vi "Grain Boundary Genie.vi"() -> ()   [LabVIEW 2010]
uses:
  <vilib>/Analysis/baseanly.llb/Real Dot Product.vi
  <vilib>/Analysis/baseanly.llb/Vector x A.vi
  <vilib>/Analysis/_algsub.llb/Real Vector Norm.vi
  <vilib>/Analysis/baseanly.llb/Real A x B.vi
  <vilib>/Utility/file.llb/Write To Spreadsheet File (string).vi
  <vilib>/Utility/file.llb/Read From Spreadsheet File (string).vi
  <vilib>/Analysis/NI_AALBase.lvlib
  <vilib>/Analysis/NI_AALPro.lvlib
  <vilib>/picture/3D Picture Control/NI_3D Picture Control.lvlib
  <vilib>/Analysis/baseanly.llb/A x Vector.vi
panel:
  in  "New Lattice Vector a 2":dbl[](array[numeric])=[6.0, 0.0, 0.0]
  in  "New Lattice Vector b 2":dbl[](array[numeric])=[0.0, 6.0, 0.0]
  in  "New Lattice Vector c 2":dbl[](array[numeric])=[0.0, 0.0, 6.0]
  out "Grain Boundary Definition":T1={"Grain 1 Orientation"=[1.0, 0.0, 0.0], "Grain 2 Orientation"=[1.0, 0.0, 0.0], "Twist Angle (Deg)"=0.0, "Translation Vector"=[0.0, 0.0, 0.0]}
  in  "Make GB":bool=TRUE
  out "STEM Viewing Angles Array":dbl[][](array[numeric])=[[0.0, 1.0, 0.0], [0.0, 0.0, 1.0], [0.0, 1.0, 1.0], [0.0, -1.0, 1.0], [0.0, 1.0, -1.0]]
  in  "Make Grain 2":bool=TRUE
  in  "Make Grain 1":bool=TRUE
  out "Grain 2 Primative":T2={"Structure Name"="CdTe", "Lattice vector a"=[0.0, 0.0, 6.615785553057252], "Lattice vector b"=[6.615785553057252, 0.0, 0.0], "Lattice vector c"=[0.0, -6.615785553057252, 0.0], "Atoms Array"=[{"Atom Name"="Cd", "Positions (Direct)"=[[0.0, 0.0, 0.0], [0.0, 0.5, 0.5], [0.5, 0.0, 0.5], [0.5, 0.5, 0.0]], "Positions (Cartesian)"=[[0.0, 0.0, 0.0], [3.307892776528626, -3.307892776528626, 0.0], [0.0, -3.307892776528626, 3.307892776528626], [3.307892776528626, 0.0, 3.307892776528626]]}, {"Atom Name"="Te", "Positions (Direct)"=[[0.25, 0.25, 0.25], [0.75, 0.75, 0.25], [0.75, 0.25, 0.75], [0.25, 0.75, 0.75]], "Positions (Cartesian)"=[[1.653946388264313, -1.653946388264313, 1.653946388264313], [4.96183916479294, -1.653946388264313, 4.96183916479294], [1.653946388264313, -4.96183916479294, 4.96183916479294], [4.96183916479294, -4.96183916479294, 1.653946388264313]]}], "# of atoms"=8} {"Atoms Array"."Positions (Cartesian)" format="%#_4f"; "Atoms Array"."Positions (Direct)" format="%#_4f"}
  in  "Load GB VESTA":bool
  in  "Load G2 VESTA":bool
  in  "Load G1 VESTA":bool
  in  "Conventional Unit Cell":T2={"Structure Name"="CdTe", "Lattice vector a"=[6.615785553057252, 0.0, 0.0], "Lattice vector b"=[0.0, 6.615785553057252, 0.0], "Lattice vector c"=[0.0, 0.0, 6.615785553057252], "Atoms Array"=[{"Atom Name"="Cd", "Positions (Direct)"=[[0.0, 0.0, 0.0], [0.0, 0.5, 0.5], [0.5, 0.0, 0.5], [0.5, 0.5, 0.0]], "Positions (Cartesian)"=[[0.0, 0.0, 0.0], [0.0, 3.307892776528626, 3.307892776528626], [3.307892776528626, 0.0, 3.307892776528626], [3.307892776528626, 3.307892776528626, 0.0]]}, {"Atom Name"="Te", "Positions (Direct)"=[[0.25, 0.25, 0.25], [0.75, 0.75, 0.25], [0.75, 0.25, 0.75], [0.25, 0.75, 0.75]], "Positions (Cartesian)"=[[1.653946388264313, 1.653946388264313, 1.653946388264313], [4.96183916479294, 4.96183916479294, 1.653946388264313], [4.96183916479294, 1.653946388264313, 4.96183916479294], [1.653946388264313, 4.96183916479294, 4.96183916479294]]}], "# of atoms"=8}
  in  "Overlap Region":dbl(slide) scale=-2.0..2.0
  in  "Tab Control":T3(tab)
  in  "GB Slider":u16(ring) items=["G1 Height", "G1 Width", "G1 Length", "G1 Start"]
  in  "GB Size Slider":dbl(slide) scale=0.0..1.0
  in  "Suggest Sizes":bool
  in  "Integer Tolerance":dbl=0.01
  in  "GB Geometric Type":T4(tab)
  in  "Use same H and W":bool=TRUE
  in  "Grain 2 Size":T5={"Height"=1.0, "Width"=1.0, "Length"=1.0, "Start"=0.0}
  in  "Grain 1 Size":T5={"Height"=1.0, "Width"=1.0, "Length"=1.0, "Start"=0.0}
  in  "Grain 2 Monoclinic size":T6={"Height"=1.0, "Width"=1.0, "Angle (deg)"=1.0, "Length"=1.0, "Start"=0.0}
  in  "Grain 1 Monoclinic size":T6={"Height"=1.0, "Width"=1.0, "Angle (deg)"=1.0, "Length"=1.0, "Start"=0.0}
  in  "Use same H, W and angle":bool=TRUE
  in  "New Lattice Vector a":dbl[](array[numeric])=[6.0, 0.0, 0.0]
  in  "New Lattice Vector c":dbl[](array[numeric])=[0.0, 0.0, 6.0]
  in  "New Lattice Vector b":dbl[](array[numeric])=[0.0, 6.0, 0.0]
  in  "Options":cluster{"Border?":bool, "Bonds?":bool}={"Border?"=TRUE, "Bonds?"=FALSE}
  in  "Zoom Scale":dbl(slide)=0.06161137440758294 scale=0.0..0.2
  in  "Mutual Viewing Angle":dbl[](array[numeric])=[0.0, 1.0, 0.0]
  in  "STEM Viewing Angles":u16(ring) items=["[0,0,1]", "[-0,-0,-1]", "[-0,0,1]", "[0,-0,1]", "[0,0,-1]", "[-0,-0,1]", "[0,-0,-1]", "[-0,0,-1]", "[-1,1,0]", "[1,-1,0]", "[1,-1,-0]", "[-1,1,-0]"]
  in  "Setup Camera":bool
  out "STEM Viewable?":bool=TRUE
  in  "Force Orthorhombic?":bool
  in  "Remove Close Atoms":bool
  in  "Crop to Smallest Repeating":bool
  in  "Slab Y":dbl=6.0
  in  "Slab X":dbl=6.0
  in  "Tolerance (A)":dbl=1.0
  in  "Minimally Allowable Distance (A)":dbl=1.5
  out "# of Atoms Removed":i32
  out "Repeating X Length Scale":dbl=99.01964045547014
  out "Subset for X?":bool
  out "Repeating Y Length Scale":dbl=99.01964045547014
  out "Subset for Y?":bool
  out "% of normal atomic density":dbl=225.0005167366452
  out "Grain 2 Integers":dbl[](array[numeric])=[1.0, 1.0, 1.0]
  out "Grain 1 Integers":dbl[](array[numeric])=[1.0, 1.0, 1.0]
  out "Misorientation Angle":dbl=60.00000000000001
  out "Suggested Viewing Angle":dbl[](array[numeric])=[-1.0, 1.0, 0.0]
  out "# of Atoms":i32=36
  out "# of Cd Atoms":i32=28
  out "# of Te Atoms":i32=8
  in  "Load GB Config":bool
  in  "Save to GB config file":bool
  in  "Structure Name":string="(60.00) twist [1.000,1.000,1.000] [1.000,1.000,1.000] (0.00,0.00,0.00)T GB"
  in  "Save to POSCAR":bool
  in  "Relaxation Type":string(combo)="conv opti"
  in  "Save into GULP":bool
  in  "Vesta .exe Location":path=path "C:/Program Files (x86)/VESTA/VESTA.exe"
  out "Lattice Parameter":dbl=6.615785553057252
  in  "Timeout Activity":string(combo)="Analyze GB"
  out "Grain Boundary Object":refnum<vi>
  out "Grain 2 Object":refnum<vi>
  out "Grain 1 Object":refnum<vi>
  in  "Add Tilt Angle":dbl(slide) scale=-5.0..15.0
  out "Grain Boundary":T2={"Structure Name"="Grain Boundary", "Lattice vector a"=[6.615785553057252, 0.0, 0.0], "Lattice vector b"=[0.0, 6.615785553057252, 0.0], "Lattice vector c"=[0.0, 0.0, 13.231571106114504], "Atoms Array"=[{"Atom Name"="Cd", "Positions (Direct)"=[[0.0, 0.0, 0.0], [0.0, 0.0, 0.5], [0.0, 0.5, 0.25], [0.0, 1.0, 0.0], [0.0, 1.0, 0.5], [0.5, 0.0, 0.25], [0.5, 0.5, 0.0], [0.5, 0.5, 0.5], [0.5, 1.0, 0.25], [1.0, 0.0, 0.0], [1.0, 0.0, 0.5], [1.0, 0.5, 0.25], [1.0, 1.0, 0.0], [1.0, 1.0, 0.5], [0.0, 0.0, 0.5], [0.0, 0.0, 1.0], [0.0, 0.5, 0.75], [0.0, 1.0, 0.5], [0.0, 1.0, 1.0], [0.5, 0.0, 0.75], [0.5, 0.5, 0.5], [0.5, 0.5, 1.0], [0.5, 1.0, 0.75], [1.0, 0.0, 0.5], [1.0, 0.0, 1.0], [1.0, 0.5, 0.75], [1.0, 1.0, 0.5], [1.0, 1.0, 1.0]], "Positions (Cartesian)"=[[0.0, 0.0, 0.0], [0.0, 0.0, 6.615785553057252], [0.0, 3.307892776528626, 3.307892776528626], [0.0, 6.615785553057252, 0.0], [0.0, 6.615785553057252, 6.615785553057252], [3.307892776528626, 0.0, 3.307892776528626], [3.307892776528626, 3.307892776528626, 0.0], [3.307892776528626, 3.307892776528626, 6.615785553057252], [3.307892776528626, 6.615785553057252, 3.307892776528626], [6.615785553057252, 0.0, 0.0], [6.615785553057252, 0.0, 6.615785553057252], [6.615785553057252, 3.307892776528626, 3.307892776528626], [6.615785553057252, 6.615785553057252, 0.0], [6.615785553057252, 6.615785553057252, 6.615785553057252], [0.0, 0.0, 6.615785553057252], [0.0, 0.0, 13.231571106114504], [0.0, 3.307892776528626, 9.92367832958588], [0.0, 6.615785553057252, 6.615785553057252], [0.0, 6.615785553057252, 13.231571106114504], [3.307892776528626, 0.0, 9.92367832958588], [3.307892776528626, 3.307892776528626, 6.615785553057252], [3.307892776528626, 3.307892776528626, 13.231571106114504], [3.307892776528626, 6.615785553057252, 9.92367832958588], [6.615785553057252, 0.0, 6.615785553057252], [6.615785553057252, 0.0, 13.231571106114504], [6.615785553057252, 3.307892776528626, 9.92367832958588], [6.615785553057252, 6.615785553057252, 6.615785553057252], [6.615785553057252, 6.615785553057252, 13.231571106114504]]}, {"Atom Name"="Te", "Positions (Direct)"=[[0.25, 0.24999999999999992, 0.375], [0.25, 0.75, 0.125], [0.75, 0.24999999999999992, 0.125], [0.75, 0.75, 0.375], [0.25, 0.24999999999999992, 0.875], [0.25, 0.75, 0.625], [0.75, 0.24999999999999992, 0.625], [0.75, 0.75, 0.875]], "Positions (Cartesian)"=[[1.653946388264313, 1.6539463882643126, 4.96183916479294], [1.653946388264313, 4.96183916479294, 1.653946388264313], [4.96183916479294, 1.6539463882643126, 1.653946388264313], [4.96183916479294, 4.96183916479294, 4.96183916479294], [1.653946388264313, 1.6539463882643126, 11.577624717850192], [1.653946388264313, 4.96183916479294, 8.269731941321565], [4.96183916479294, 1.6539463882643126, 8.269731941321565], [4.96183916479294, 4.96183916479294, 11.577624717850192]]}], "# of atoms"=36} {"Atoms Array"."Positions (Cartesian)" format="%#_4f"; "Atoms Array"."Positions (Direct)" format="%#_4f"}
  out "Grain 2":T2={"Structure Name"="CdTe Expanded to Box", "Lattice vector a"=[6.615785553057252, 0.0, 0.0], "Lattice vector b"=[0.0, 6.615785553057252, 0.0], "Lattice vector c"=[0.0, 0.0, 6.615785553057252], "Atoms Array"=[{"Atom Name"="Cd", "Positions (Direct)"=[[0.0, 0.0, 0.0], [0.0, 0.0, 1.0], [0.0, 0.5, 0.5], [0.0, 1.0, 0.0], [0.0, 1.0, 1.0], [0.5, 0.0, 0.5], [0.5, 0.5, 0.0], [0.5, 0.5, 1.0], [0.5, 1.0, 0.5], [1.0, 0.0, 0.0], [1.0, 0.0, 1.0], [1.0, 0.5, 0.5], [1.0, 1.0, 0.0], [1.0, 1.0, 1.0]], "Positions (Cartesian)"=[[0.0, 0.0, 0.0], [0.0, 0.0, 6.615785553057252], [0.0, 3.307892776528626, 3.307892776528626], [0.0, 6.615785553057252, 0.0], [0.0, 6.615785553057252, 6.615785553057252], [3.307892776528626, 0.0, 3.307892776528626], [3.307892776528626, 3.307892776528626, 0.0], [3.307892776528626, 3.307892776528626, 6.615785553057252], [3.307892776528626, 6.615785553057252, 3.307892776528626], [6.615785553057252, 0.0, 0.0], [6.615785553057252, 0.0, 6.615785553057252], [6.615785553057252, 3.307892776528626, 3.307892776528626], [6.615785553057252, 6.615785553057252, 0.0], [6.615785553057252, 6.615785553057252, 6.615785553057252]]}, {"Atom Name"="Te", "Positions (Direct)"=[[0.25, 0.24999999999999992, 0.75], [0.25, 0.75, 0.25], [0.75, 0.24999999999999992, 0.25], [0.75, 0.75, 0.75]], "Positions (Cartesian)"=[[1.653946388264313, 1.6539463882643126, 4.96183916479294], [1.653946388264313, 4.96183916479294, 1.653946388264313], [4.96183916479294, 1.6539463882643126, 1.653946388264313], [4.96183916479294, 4.96183916479294, 4.96183916479294]]}], "# of atoms"=18} {"Atoms Array"."Positions (Cartesian)" format="%#_4f"; "Atoms Array"."Positions (Direct)" format="%#_4f"}
  out "Grain 1":T2={"Structure Name"="CdTe Expanded to Box", "Lattice vector a"=[6.615785553057252, 0.0, 0.0], "Lattice vector b"=[0.0, 6.615785553057252, 0.0], "Lattice vector c"=[0.0, 0.0, 6.615785553057252], "Atoms Array"=[{"Atom Name"="Cd", "Positions (Direct)"=[[0.0, 0.0, 0.0], [0.0, 0.0, 1.0], [0.0, 0.5, 0.5], [0.0, 1.0, 0.0], [0.0, 1.0, 1.0], [0.5, 0.0, 0.5], [0.5, 0.5, 0.0], [0.5, 0.5, 1.0], [0.5, 1.0, 0.5], [1.0, 0.0, 0.0], [1.0, 0.0, 1.0], [1.0, 0.5, 0.5], [1.0, 1.0, 0.0], [1.0, 1.0, 1.0]], "Positions (Cartesian)"=[[0.0, 0.0, 0.0], [0.0, 0.0, 6.615785553057252], [0.0, 3.307892776528626, 3.307892776528626], [0.0, 6.615785553057252, 0.0], [0.0, 6.615785553057252, 6.615785553057252], [3.307892776528626, 0.0, 3.307892776528626], [3.307892776528626, 3.307892776528626, 0.0], [3.307892776528626, 3.307892776528626, 6.615785553057252], [3.307892776528626, 6.615785553057252, 3.307892776528626], [6.615785553057252, 0.0, 0.0], [6.615785553057252, 0.0, 6.615785553057252], [6.615785553057252, 3.307892776528626, 3.307892776528626], [6.615785553057252, 6.615785553057252, 0.0], [6.615785553057252, 6.615785553057252, 6.615785553057252]]}, {"Atom Name"="Te", "Positions (Direct)"=[[0.25, 0.24999999999999992, 0.75], [0.25, 0.75, 0.25], [0.75, 0.24999999999999992, 0.25], [0.75, 0.75, 0.75]], "Positions (Cartesian)"=[[1.653946388264313, 1.6539463882643126, 4.96183916479294], [1.653946388264313, 4.96183916479294, 1.653946388264313], [4.96183916479294, 1.6539463882643126, 1.653946388264313], [4.96183916479294, 4.96183916479294, 4.96183916479294]]}], "# of atoms"=18} {"Atoms Array"."Positions (Cartesian)" format="%#_4f"; "Atoms Array"."Positions (Direct)" format="%#_4f"}
  in  "Primitive Lattice Vectors":T2={"Structure Name"="Relax2 Subcrystal", "Lattice vector a"=[0.0, 3.3046962263585, 3.3046962263585], "Lattice vector b"=[3.3046962263585, 0.0, 3.3046962263585], "Lattice vector c"=[3.3046962263585, 3.3046962263585, 0.0], "Atoms Array"=[{"Atom Name"="Cd", "Positions (Direct)"=[[0.0, 0.0, 0.0]], "Positions (Cartesian)"=[[0.0, 0.0, 0.0]]}, {"Atom Name"="Te", "Positions (Direct)"=[[0.25, 0.25, 0.25]], "Positions (Cartesian)"=[[1.65234811317925, 1.65234811317925, 1.65234811317925]]}], "# of atoms"=2} {"Atoms Array"."Positions (Cartesian)" format="%#_4f"; "Atoms Array"."Positions (Direct)" format="%#_4f"}
  out "Grain Boundary Render":refnum<vi>(3d-picture)
  in  "Translation Vector":dbl[](array[slide])=[0.0, 0.0, 0.0] scale=0.0..4.0
  in  "Twist Angle":dbl(slide) scale=0.0..38.0
  in  "Grain 2 Orientation":dbl[](array[numeric])=[1.0, 0.0, 0.0]
  in  "Grain 1 Orientation":dbl[](array[numeric])=[1.0, 0.0, 0.0]
  out "Grain 2 Render":refnum<vi>(3d-picture)
  out "Grain 1 Render":refnum<vi>(3d-picture)
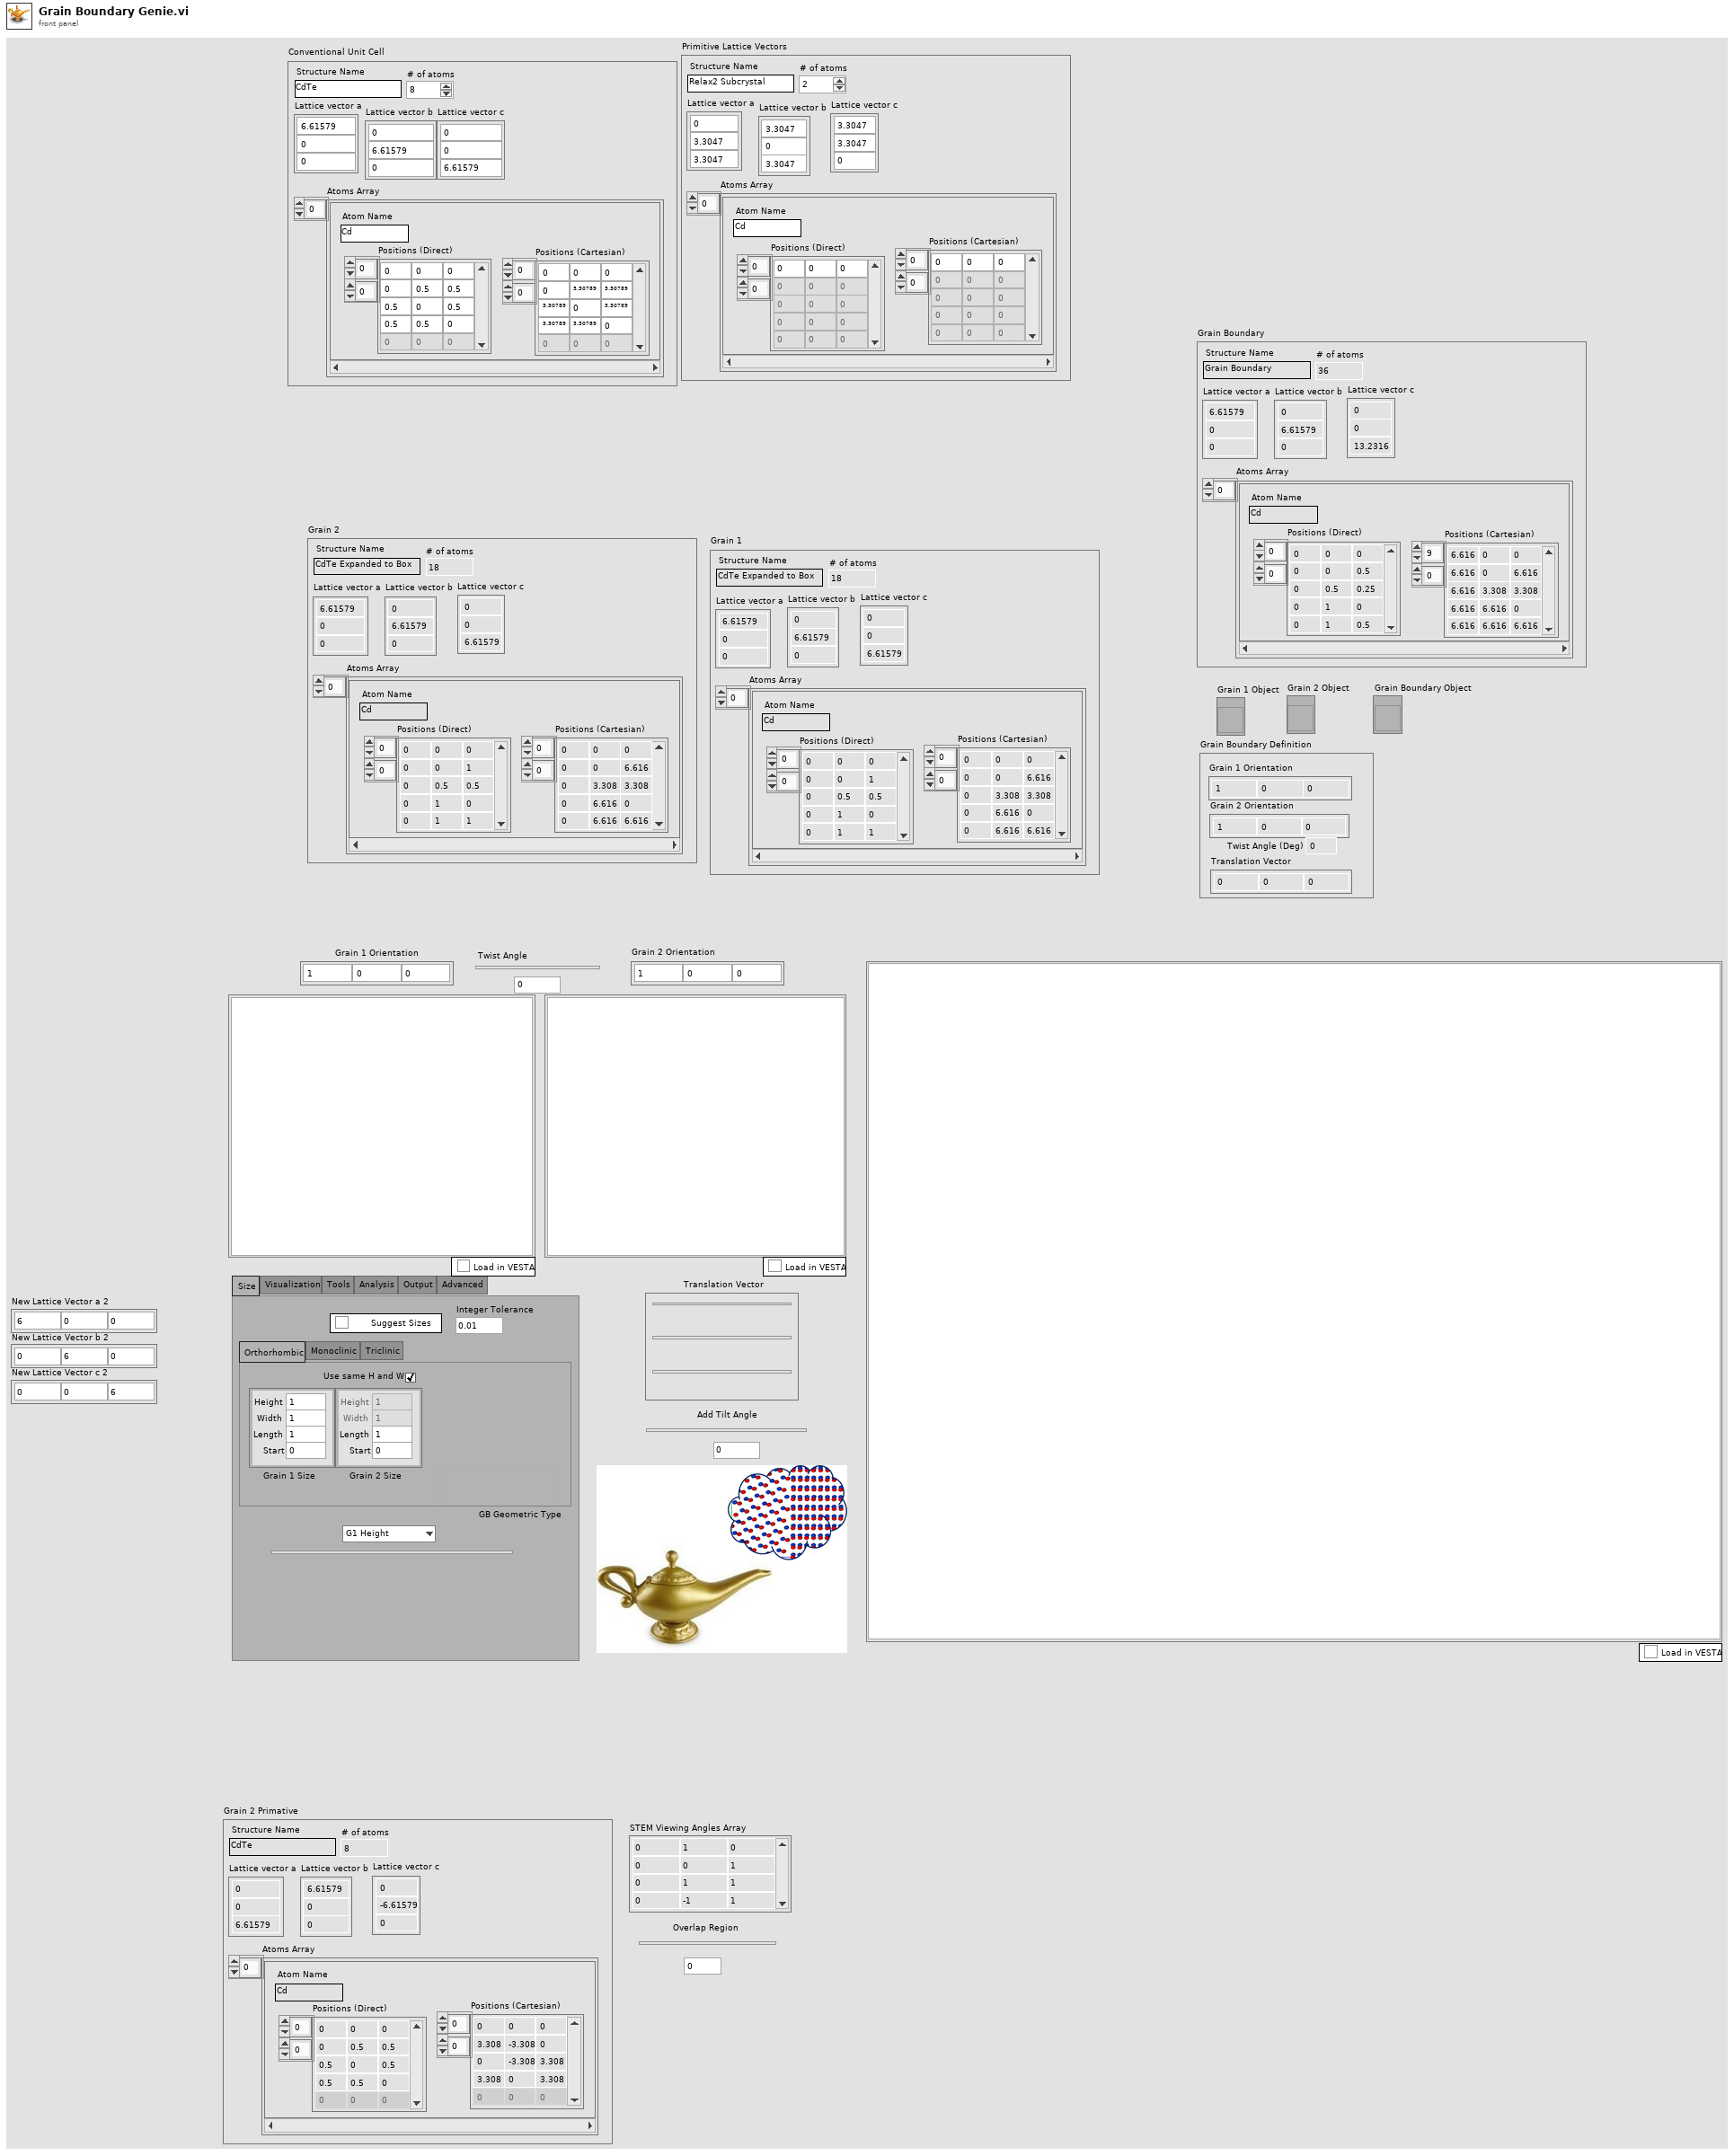
[diagram p1: front panel]
types:
  T1 = cluster{"Grain 1 Orientation":dbl[], "Grain 2 Orientation":dbl[], "Twist Angle (Deg)":dbl, "Translation Vector":dbl[]}
  T2 = cluster{"Structure Name":string, "Lattice vector a":dbl[], "Lattice vector b":dbl[], "Lattice vector c":dbl[], "Atoms Array":cluster{"Atom Name":string, "Positions (Direct)":dbl[][], "Positions (Cartesian)":dbl[][]}[], "# of atoms":i32}
  T3 = enum32{"Size", "Visualization", "Tools", "Analysis", "Output", "Advanced"}
  T4 = enum32{"Orthorhombic", "Monoclinic", "Triclinic"}
  T5 = cluster{"Height":dbl, "Width":dbl, "Length":dbl, "Start":dbl}
  T6 = cluster{"Height":dbl, "Width":dbl, "Angle (deg)":dbl, "Length":dbl, "Start":dbl}
  T7 = enum8{"Enabled", "Disabled", "Disabled and Grayed Out"}
  T8 = cluster{"Atom Name":string, "Positions (Direct)":dbl[][], "Positions (Cartesian)":dbl[][]}[]
  T9 = typedef "NI_Matrix.lvlib/RealMatrix.ctl" = dbl[][]
  T10 = cluster{"Misorientation Angle":dbl, "Misorientation Axis, o":dbl[], "Misorientation Matrix":T9}
  T11 = cluster{"Atom Name":string, "Positions (Direct)":dbl[][], "Positions (Cartesian)":dbl[][]}
  T12 = cluster{"Grain 1 Orientation":dbl[], "Grain 2 Orientation":dbl[], "Twist Angle":dbl, "Translation Vector":dbl[]}
  T13 = cluster{"Z Min":dbl, "Width":dbl, "Z Min":dbl, "Height":dbl, "Start":dbl, "Length":dbl}
  T14 = cluster{"Z Min":dbl, dbl, "Z Min":dbl, dbl, "Start":dbl, "Length":dbl}
  T15 = cluster{"Z Min":dbl, dbl, "Z Min":dbl, dbl, "Z Min":dbl, dbl}
  T16 = cluster{"Z Min":dbl, "Width":dbl, "Z Min":dbl, dbl, "Start":dbl, "Length":dbl}
  T17 = cluster{"String":dbl, "String":dbl, "String":dbl, "String":dbl}
  T18 = cluster{"Grain 1 Orientation":dbl[], "Grain 2 Orientation":dbl[], "Twist Angle":dbl}
  T19 = cluster{"Grain 1 Length (prop)":dbl, "Grain 2 Length (prop)":dbl, "Grain 1 Height (prop)":dbl, "Grain 2 Height (prop)":dbl, "Grain 1 Width (prop)":dbl, "Grain 2 Width (prop)":dbl}
  T20 = cluster{"Grain 1 Height (prop)":dbl, "Grain 1 Width (prop)":dbl, "Grain 1 Length (prop)":dbl, "y":dbl}
  T21 = cluster{"Grain 2 Height (prop)":dbl, "Grain 2 Width (prop)":dbl, "Grain 2 Length (prop)":dbl, "y":dbl}
  T22 = cluster{"[0]":dbl, "[1]":dbl, "[2]":dbl, "[3]":dbl}
  T23 = cluster{"[0]":dbl, "[1]":dbl, "[2]":dbl, "[3]":dbl, "[4]":dbl}
  T24 = cluster{"Lattice vector b[0]":dbl, "Lattice vector b[1]":dbl, "Lattice vector b[2]":dbl}
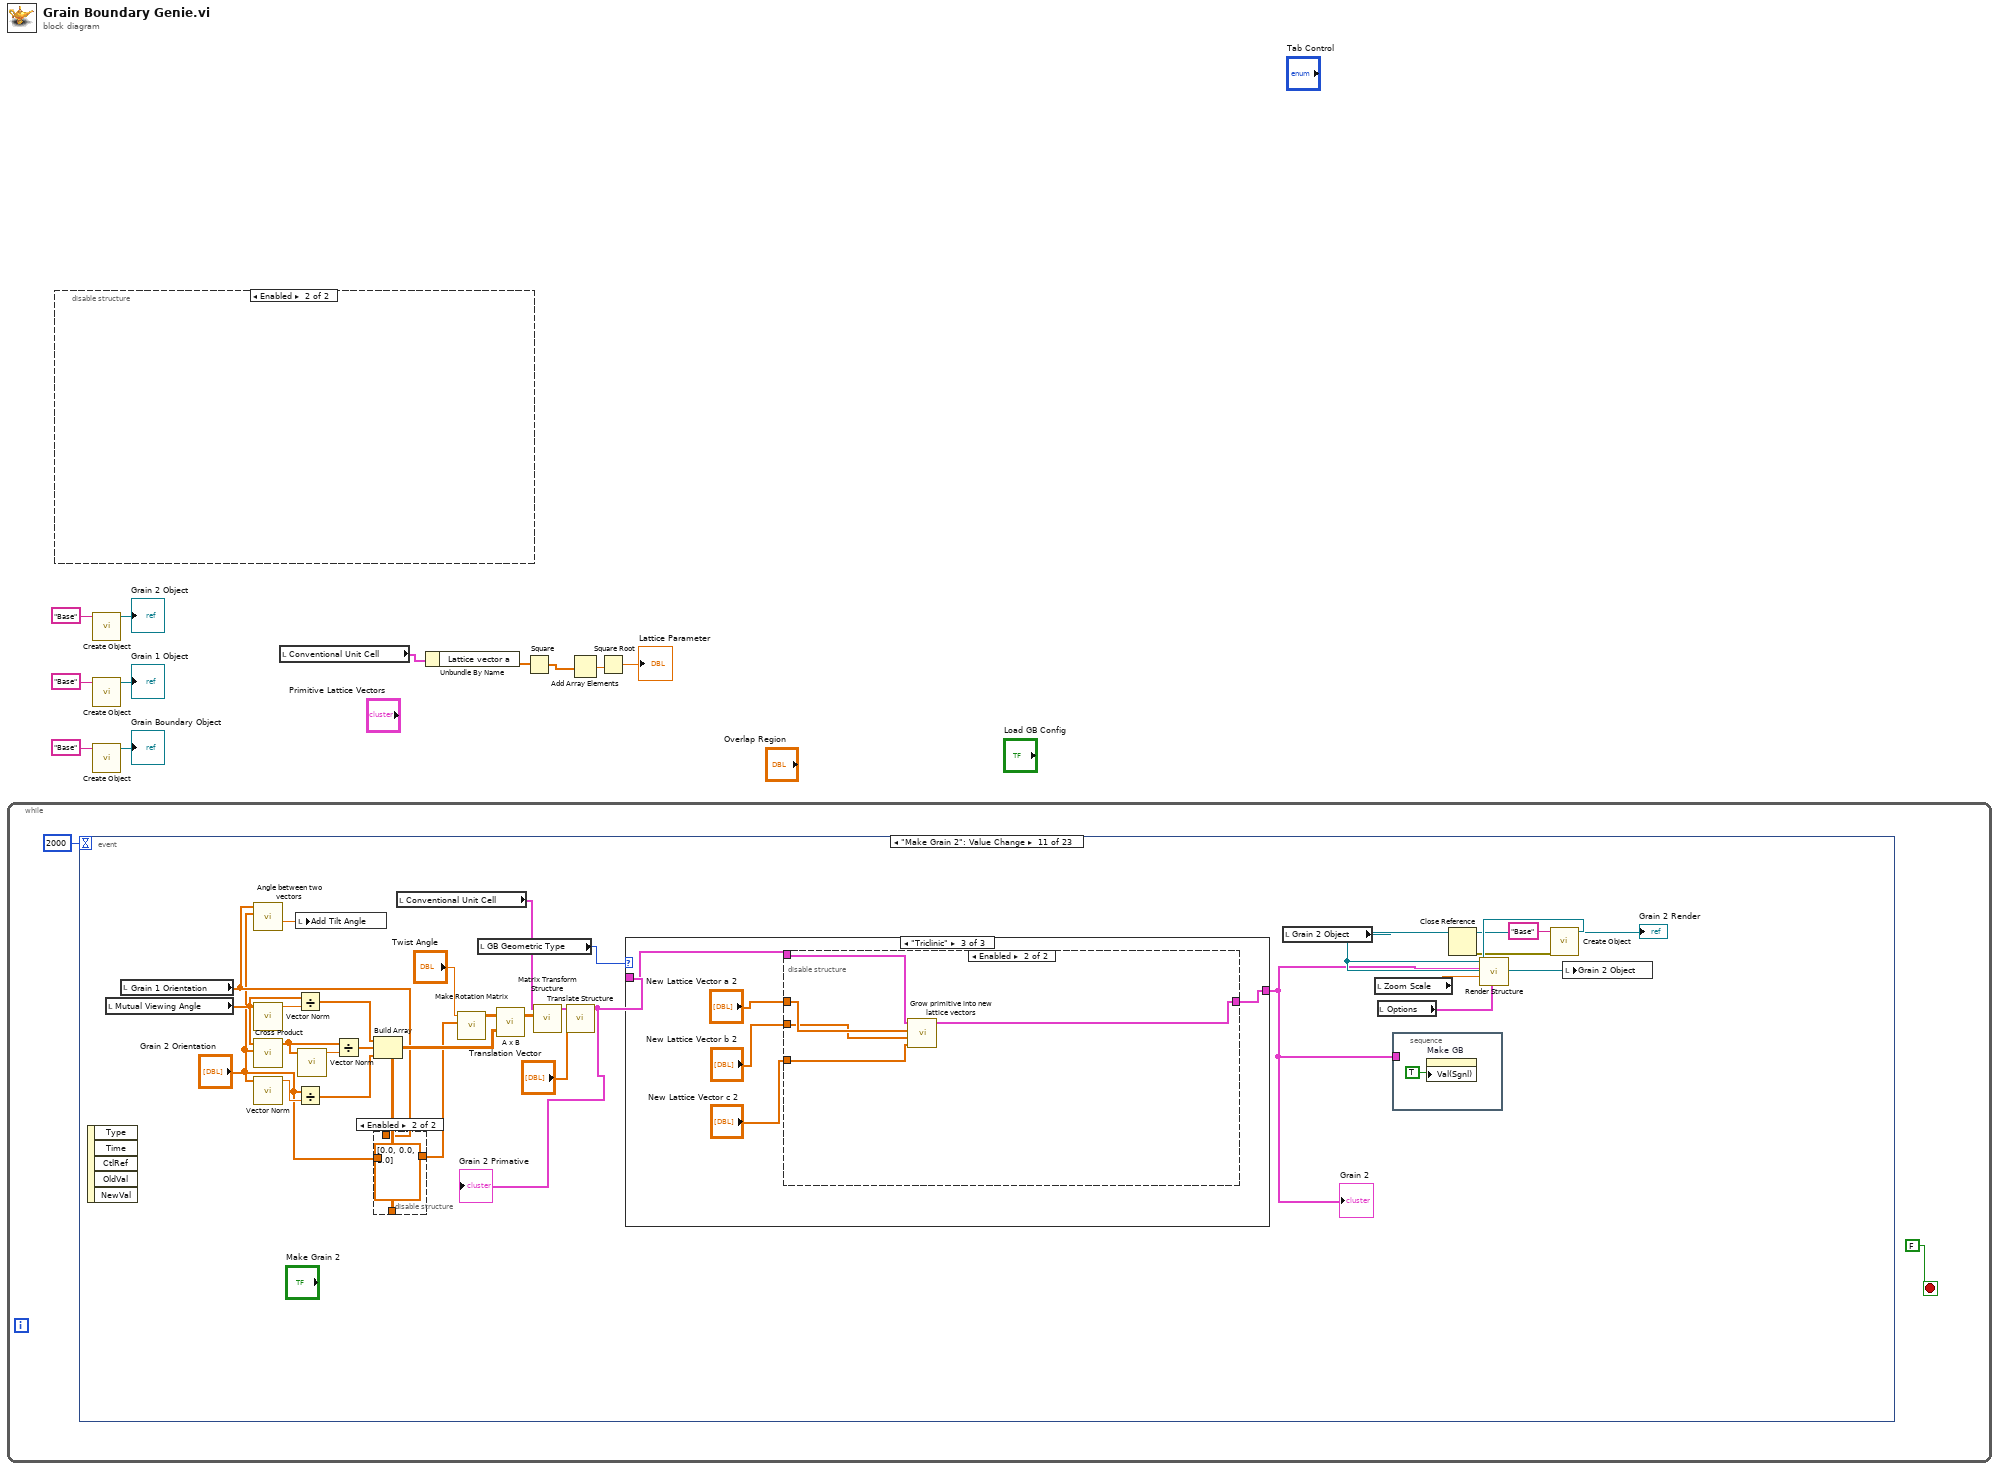
[diagram p0: block diagram]
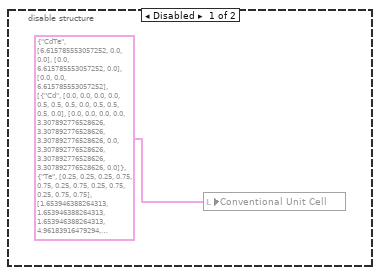
[diagram p2: hidden frame]
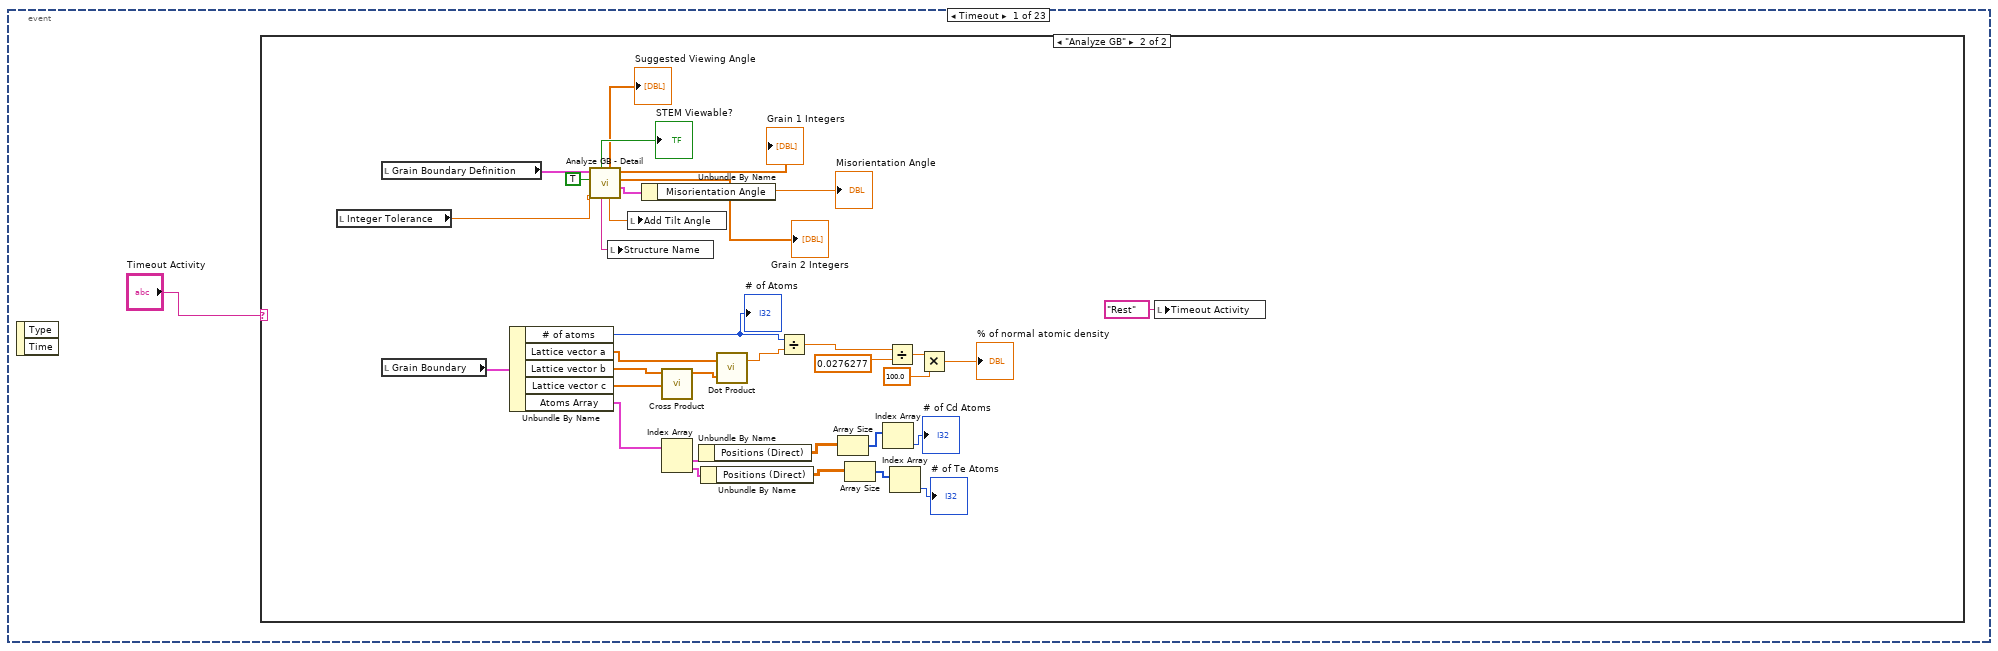
[diagram p3: hidden frame]
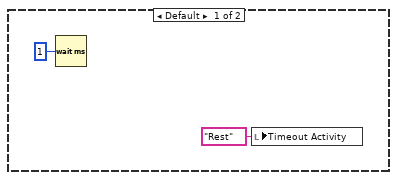
[diagram p4: hidden frame]
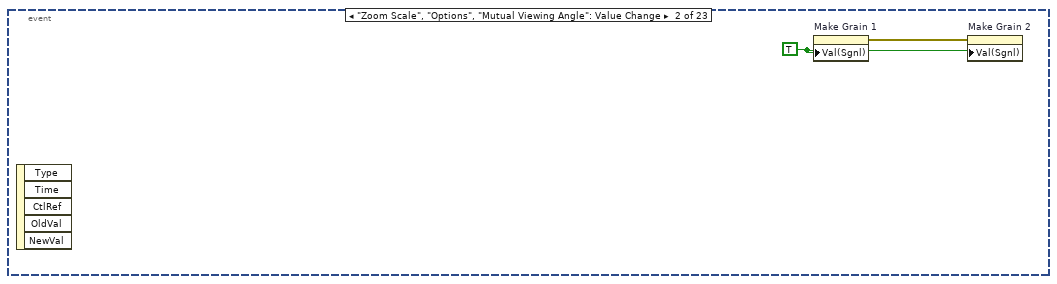
[diagram p5: hidden frame]
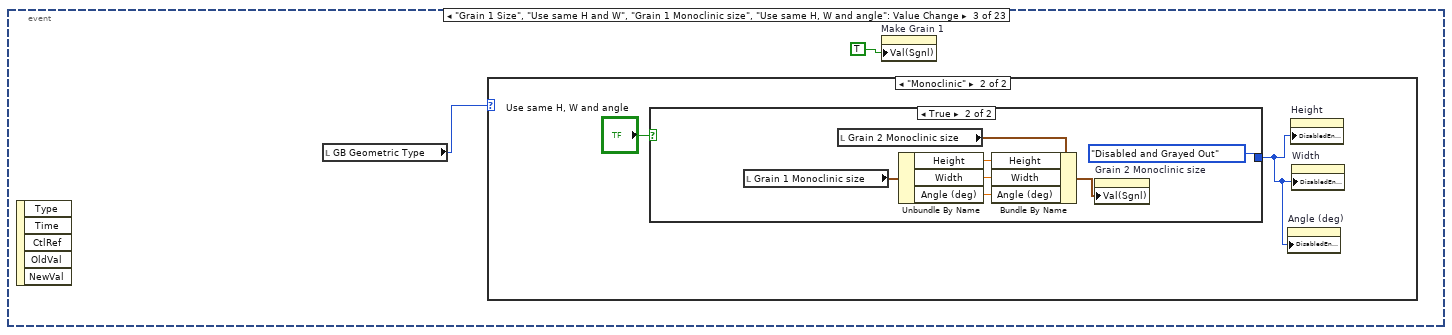
[diagram p6: hidden frame]
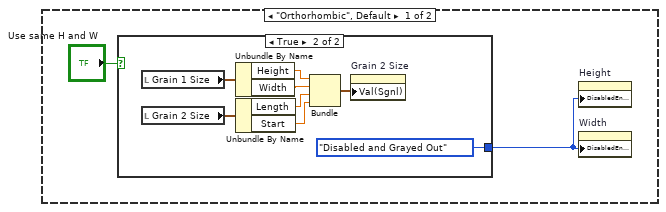
[diagram p7: hidden frame]
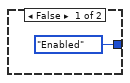
[diagram p8: hidden frame]
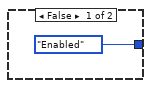
[diagram p9: hidden frame]
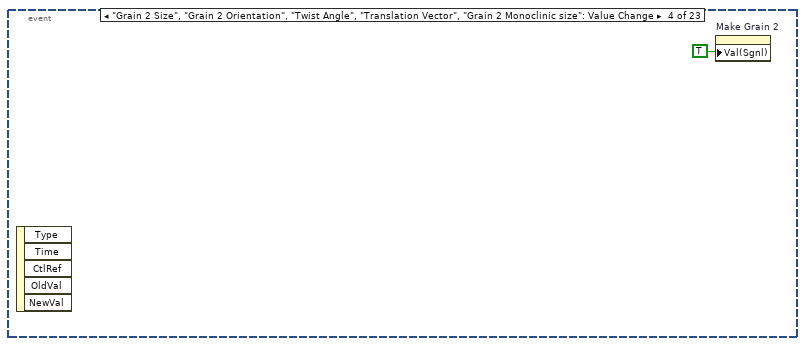
[diagram p10: hidden frame]
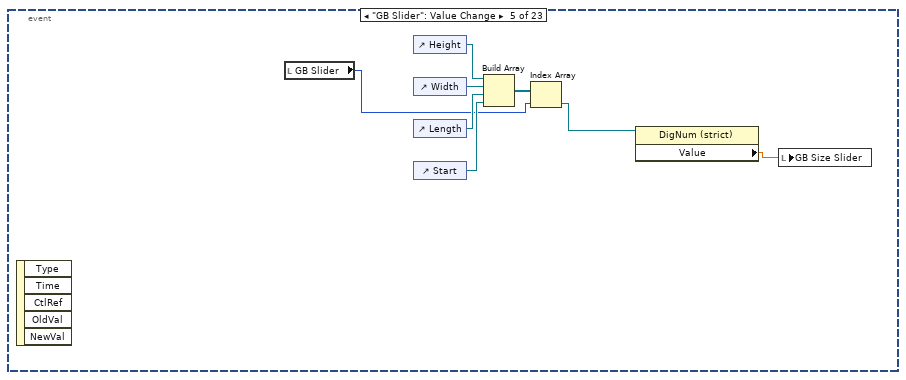
[diagram p11: hidden frame]
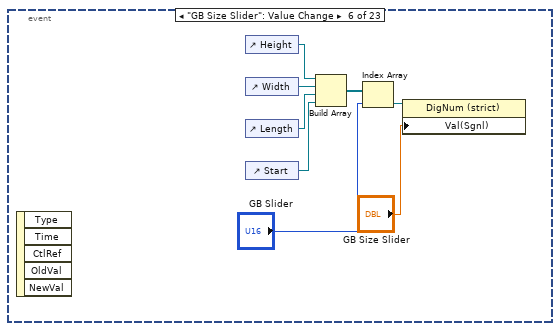
[diagram p12: hidden frame]
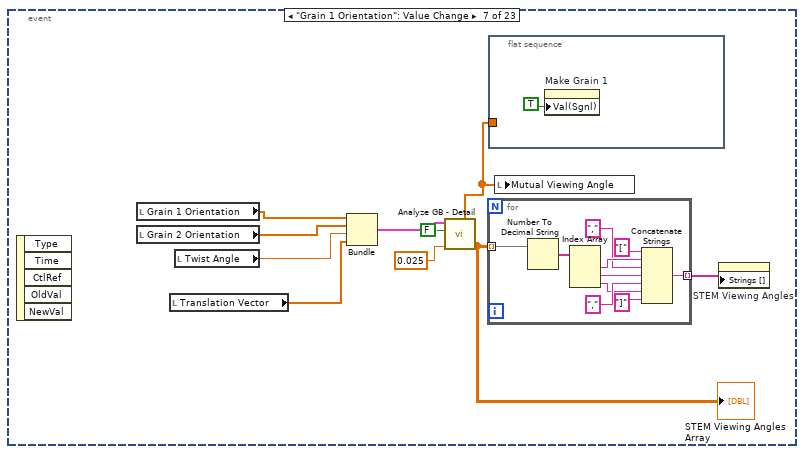
[diagram p13: hidden frame]
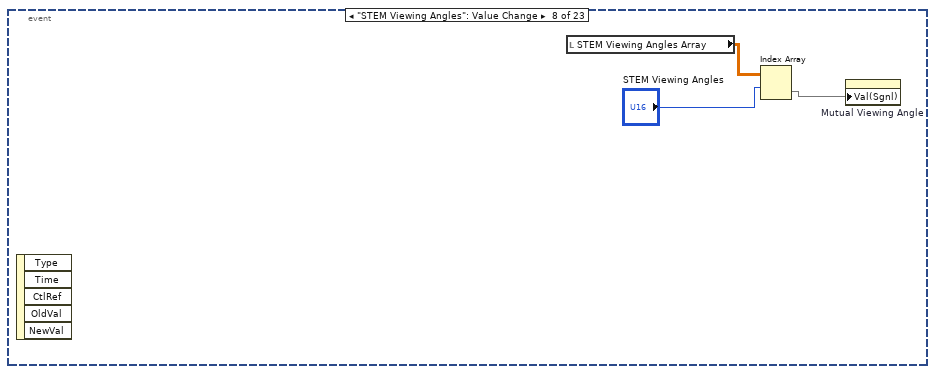
[diagram p14: hidden frame]
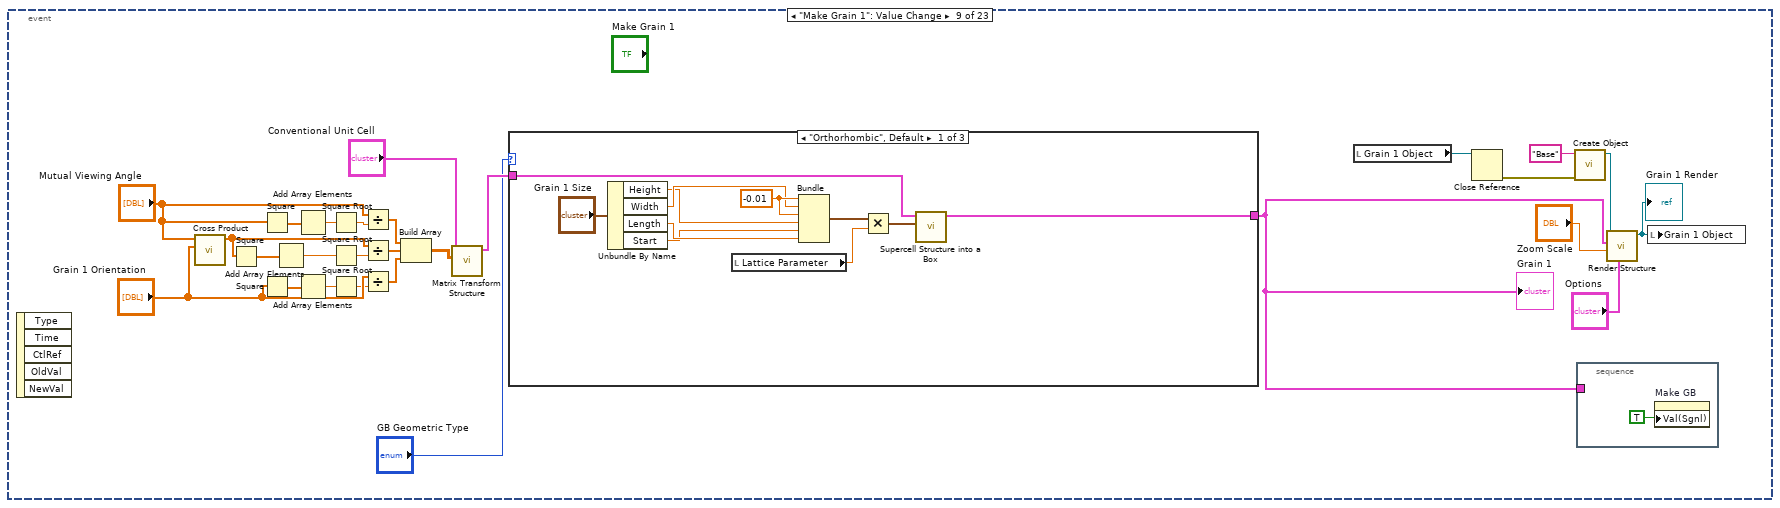
[diagram p15: hidden frame]
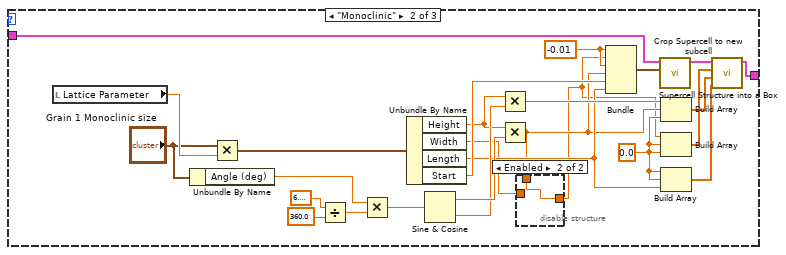
[diagram p16: hidden frame]
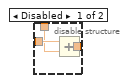
[diagram p17: hidden frame]
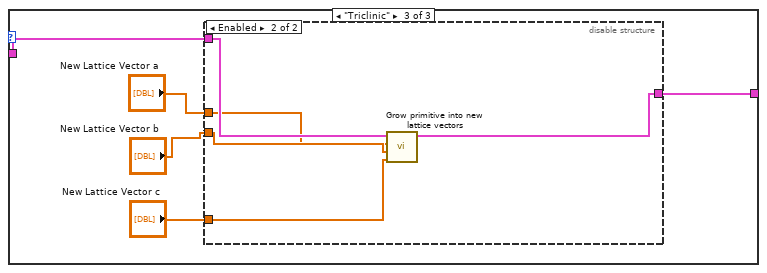
[diagram p18: hidden frame]
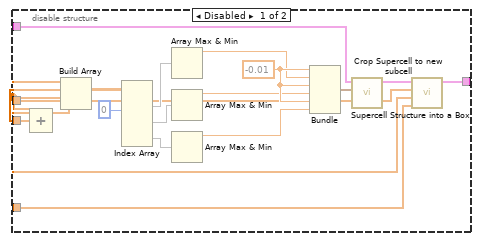
[diagram p19: hidden frame]
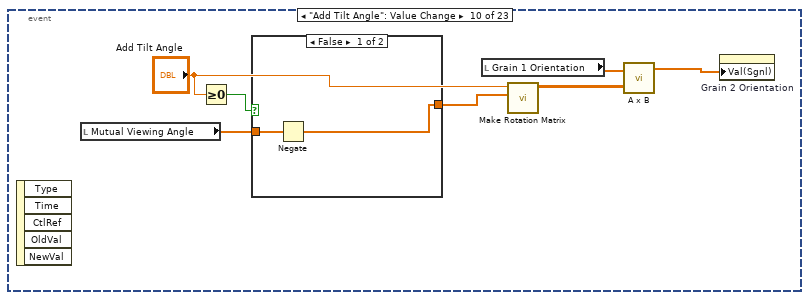
[diagram p20: hidden frame]
diagram:
  n1 = while {
    stop <- FALSE stop-if-true
    n2 = event shown="[10] \"Make Grain 2\": Value Change" {
      selector: _ -> [_ _ _ _ _ _ _ _ _ _ _ _ _ _ _ _ _ _ _ _ _ _ _]
      dyn-events: _ -> [_ _ _ _ _ _ _ _ _ _ _ _ _ _ _ _ _ _ _ _ _ _ _]
      timeout: 2000 -> [_ _ _ _ _ _ _ _ _ _ _ _ _ _ _ _ _ _ _ _ _ _ _]
      event Timeout {
        n3 = event-data() -> ()  [unwired: 1 in, 2 out]
        n4 = case shown="\"Analyze GB\"" "Timeout Activity" {
          frame Default {
            n5 = Wait (ms)(milliseconds to wait=u32 1) -> ()  [unwired: 1 out]
            n6 = local write "Timeout Activity"("Rest" ("Timeout Activity")) -> ()
          }
          frame "Analyze GB" {
            n7 = local read "Integer Tolerance"() -> (w21:dbl)
            n8 = local read "Grain Boundary Definition"() -> (w49:T1)
            n9 = local read "Grain Boundary"() -> (w23:T2)
            n10 = Unbundle By Name(w23) -> ("# of atoms"=w24:i32, "Lattice vector a"=w31:dbl[], "Lattice vector b"=w30:dbl[], "Lattice vector c"=w29:dbl[], "Atoms Array"=w22:T8)
            "# of Atoms" <- w24
            n11 = call "Analyze GB - Detail.vi"("Integer Tolerance"=w21, "Find Integer Rep?"=TRUE, "Grain Boundary Definition"=w49) -> ("Misorientation"=w35:T10, "Grain 2 Integers"=→"Grain 2 Integers":dbl[], "Grain 1 Integers"=→"Grain 1 Integers":dbl[], "Tilt Angle (Deg)"=w38:dbl, "Suggested view direction"=→"Suggested Viewing Angle":dbl[], "GB Name"=w39:string, "STEM Viewable?"=→"STEM Viewable?":bool)  [unwired: 1 in, 1 out]
            n12 = local write "Structure Name"(w39) -> ()
            n13 = local write "Add Tilt Angle"(w38) -> ()
            n14 = Unbundle By Name(w35) -> ("Misorientation Angle"=→"Misorientation Angle":dbl)
            n15 = call <vilib>:"Cross Product.vi"("B Vector"=w29, "A Vector"=w30) -> ("Cross Product"=w28:dbl[])  [unwired: 8 in, 1 out]
            n16 = Index Array(array=w22) -> (element #1=w48:T11, element #2=w47:T11)  [unwired: 2 in]
            n17 = Unbundle By Name(w48) -> ("Positions (Direct)"=w46:dbl[][])
            n18 = Unbundle By Name(w47) -> ("Positions (Direct)"=w45:dbl[][])
            n19 = call-poly <vilib>:"Dot Product.vi"("Y Vector"=w28, "X Vector"=w31) -> ("X * Y"=w27:dbl)  [unwired: 1 out]
            n20 = Divide(x=w24, y=w27) -> (x/y=w26:dbl)
            n21 = Array Size(array=w46) -> (size(s)=w44:i32[])
            n22 = Array Size(array=w45) -> (size(s)=w43:i32[])
            n23 = Index Array(array=w44) -> (element=→"# of Cd Atoms":i32)  [unwired: 1 in]
            n24 = Divide(x=w26, y=0.0276277) -> (x/y=w19:dbl)
            n25 = Index Array(array=w43) -> (element=→"# of Te Atoms":i32)  [unwired: 1 in]
            n26 = Multiply(x=w19, y=100.0) -> (x*y=→"% of normal atomic density":dbl)
            n27 = local write "Timeout Activity"("Rest" ("Timeout Activity")) -> ()
          }
        }
      }
      event "Zoom Scale", "Options", "Mutual Viewing Angle": Value Change {
        w51 = TRUE ("Value (Signaling)")
        n28 = event-data() -> ()  [unwired: 1 in, 5 out]
        n29 = property on="Make Grain 1" class="Bool (strict)"("Val(Sgnl)"=w51) -> (error out=w50:errorcluster)  [unwired: 2 in, 1 out]
        n30 = property on="Make Grain 2" class="Bool (strict)"(error in=w50, "Val(Sgnl)"=w51) -> ()  [unwired: 1 in, 2 out]
      }
      event "Grain 1 Size", "Use same H and W", "Grain 1 Monoclinic size", "Use same H, W and angle": Value Change {
        n31 = event-data() -> ()  [unwired: 1 in, 5 out]
        n32 = local read "GB Geometric Type"() -> (w52:T4)
        n33 = case shown="\"Monoclinic\"" w52 {
          frame "Orthorhombic", Default {
            n34 = case shown="True" "Use same H and W" {
              tunnel: [T7."Enabled" ("Disabled") T7."Disabled and Grayed Out" ("Disabled")] -> w54
              frame False {
              }
              frame True {
                n35 = local read "Grain 1 Size"() -> (w64:T5)
                n36 = local read "Grain 2 Size"() -> (w61:T5)
                n37 = Unbundle By Name(w64) -> ("Height"=w63:dbl, "Width"=w62:dbl)
                n38 = Unbundle By Name(w61) -> ("Length"=w60:dbl, "Start"=w59:dbl)
                n39 = Bundle("Height"=w63, "Width"=w62, "Length"=w60, "Start"=w59) -> (w58:T5)  [unwired: 1 in]
                n40 = property on="Grain 2 Size" class="Clust (strict)"("Val(Sgnl)"=w58) -> ()  [unwired: 2 in, 2 out]
              }
            }
            n41 = property on="Height" class="DigNum (strict)"("DisabledEnum"=w54) -> ()  [unwired: 2 in, 2 out]
            n42 = property on="Width" class="DigNum (strict)"("DisabledEnum"=w54) -> ()  [unwired: 2 in, 2 out]
          }
          frame "Monoclinic" {
            n43 = case shown="True" "Use same H, W and angle" {
              tunnel: [T7."Enabled" ("Disabled") T7."Disabled and Grayed Out" ("Disabled")] -> w65
              frame False {
              }
              frame True {
                n44 = local read "Grain 1 Monoclinic size"() -> (w74:T6)
                n45 = local read "Grain 2 Monoclinic size"() -> (w73:T6)
                n46 = Unbundle By Name(w74) -> ("Height"=w72:dbl, "Width"=w71:dbl, "Angle (deg)"=w70:dbl)
                n47 = Bundle By Name(cluster=w73, "Height"=w72, "Width"=w71, "Angle (deg)"=w70) -> (w69:T6)
                n48 = property on="Grain 2 Monoclinic size" class="Clust (strict)"("Val(Sgnl)"=w69) -> ()  [unwired: 2 in, 2 out]
              }
            }
            n49 = property on="Angle (deg)" class="DigNum (strict)"("DisabledEnum"=w65) -> ()  [unwired: 2 in, 2 out]
            n50 = property on="Height" class="DigNum (strict)"("DisabledEnum"=w65) -> ()  [unwired: 2 in, 2 out]
            n51 = property on="Width" class="DigNum (strict)"("DisabledEnum"=w65) -> ()  [unwired: 2 in, 2 out]
          }
        }
        n52 = property on="Make Grain 1" class="Bool (strict)"("Val(Sgnl)"=TRUE ("Value (Signaling)")) -> ()  [unwired: 2 in, 2 out]
      }
      event "Grain 2 Size", "Grain 2 Orientation", "Twist Angle", "Translation Vector", "Grain 2 Monoclinic size": Value Change {
        n53 = event-data() -> ()  [unwired: 1 in, 5 out]
        n54 = property on="Make Grain 2" class="Bool (strict)"("Val(Sgnl)"=TRUE ("Value (Signaling)")) -> ()  [unwired: 2 in, 2 out]
      }
      event "GB Slider": Value Change {
        n55 = event-data() -> ()  [unwired: 1 in, 5 out]
        n56 = local read "GB Slider"() -> (w78:u16)
        n57 = control-ref of="Height"() -> (w83:refnum<vi>)
        n58 = control-ref of="Width"() -> (w81:refnum<vi>)
        n59 = control-ref of="Length"() -> (w80:refnum<vi>)
        n60 = control-ref of="Start"() -> (w79:refnum<vi>)
        n61 = Build Array(w83, w81, w80, w79) -> (w82:refnum<vi>[])
        n62 = Index Array(array=w82, index=w78) -> (element=w77:refnum<vi>)
        n63 = property on="Property Node" class="DigNum (strict)"(reference=w77) -> ("Value"=w76:dbl)  [unwired: 1 in, 2 out]
        n64 = local write "GB Size Slider"(w76) -> ()
      }
      event "GB Size Slider": Value Change {
        n65 = event-data() -> ()  [unwired: 1 in, 5 out]
        n66 = control-ref of="Height"() -> (w89:refnum<vi>)
        n67 = control-ref of="Width"() -> (w86:refnum<vi>)
        n68 = control-ref of="Length"() -> (w85:refnum<vi>)
        n69 = control-ref of="Start"() -> (w84:refnum<vi>)
        n70 = Build Array(w89, w86, w85, w84) -> (w88:refnum<vi>[])
        n71 = Index Array(array=w88, index="GB Slider") -> (element=w87:refnum<vi>)
        n72 = property on="Property Node" class="DigNum (strict)"(reference=w87, "Val(Sgnl)"="GB Size Slider") -> ()  [unwired: 1 in, 2 out]
      }
      event "Grain 1 Orientation": Value Change {
        n73 = event-data() -> ()  [unwired: 1 in, 5 out]
        n74 = local read "Grain 1 Orientation"() -> (w97:dbl[])
        n75 = local read "Grain 2 Orientation"() -> (w96:dbl[])
        n76 = local read "Translation Vector"() -> (w94:dbl[])
        n77 = local read "Twist Angle"() -> (w95:dbl)
        n78 = Bundle("Grain 1 Orientation"=w97, "Grain 2 Orientation"=w96, "Twist Angle"=w95, "Translation Vector"=w94) -> (w93:T12)  [unwired: 1 in]
        n79 = call "Analyze GB - Detail.vi"("Integer Tolerance"=0.025, "Find Integer Rep?"=FALSE, "Grain Boundary Definition"=w93) -> ("STEM Viewing Angles"=w99:dbl[][], "Suggested view direction"=w100:dbl[])  [unwired: 1 in, 6 out]
        "STEM Viewing Angles Array" <- w99
        n80 = for {
          tunnel: w99 -> [w111] mode=indexing
          tunnel: [w102] -> w98 mode=indexing
          n81 = Number To Decimal String(number=w111) -> (decimal integer string=w110:string[])  [unwired: 1 in]
          n82 = Index Array(array=w110) -> (element #1=w108:string, element #2=w106:string, element #3=w104:string)  [unwired: 3 in]
          n83 = Concatenate Strings("[" ("string"), w108, "," ("string"), w106, "," ("string"), w104, "]" ("string")) -> (w102:string)
        }
        n84 = flat-sequence {
          tunnel: w100 -> [_]
          frame #0 {
            n85 = property on="Make Grain 1" class="Bool (strict)"("Val(Sgnl)"=TRUE ("Value (Signaling)")) -> ()  [unwired: 2 in, 2 out]
          }
        }
        n86 = local write "Mutual Viewing Angle"(w100) -> ()
        n87 = property on="STEM Viewing Angles" class="Ring (strict)"("Strings []"=w98) -> ()  [unwired: 2 in, 2 out]
      }
      event "STEM Viewing Angles": Value Change {
        n88 = event-data() -> ()  [unwired: 1 in, 5 out]
        n89 = local read "STEM Viewing Angles Array"() -> (w115:dbl[][])
        n90 = Index Array(array=w115, index (row)="STEM Viewing Angles") -> (element=w113:dbl[])  [unwired: 1 in]
        n91 = property on="Mutual Viewing Angle" class="Arr (strict)"("Val(Sgnl)"=w113) -> ()  [unwired: 2 in, 2 out]
      }
      event "Make Grain 1": Value Change {
        n92 = event-data() -> ()  [unwired: 1 in, 5 out]
        n93 = call <vilib>:"Cross Product.vi"("B Vector"="Grain 1 Orientation", "A Vector"="Mutual Viewing Angle") -> ("Cross Product"=w118:dbl[])  [unwired: 8 in, 1 out]
        n94 = Square(x=w118) -> (x^2=w119:dbl[])
        n95 = Square(x="Mutual Viewing Angle") -> (x^2=w123:dbl[])
        n96 = Square(x="Grain 1 Orientation") -> (x^2=w126:dbl[])
        n97 = Add Array Elements(numeric array=w119) -> (sum=w117:dbl)
        n98 = Add Array Elements(numeric array=w123) -> (sum=w122:dbl)
        n99 = Add Array Elements(numeric array=w126) -> (sum=w127:dbl)
        n100 = Square Root(x=w122) -> (sqrt(x)=w120:dbl)
        n101 = Square Root(x=w117) -> (sqrt(x)=w116:dbl)
        n102 = Square Root(x=w127) -> (sqrt(x)=w124:dbl)
        n103 = Divide(x="Mutual Viewing Angle", y=w120) -> (x/y=w142:dbl[])
        n104 = Divide(x=w118, y=w116) -> (x/y=w132:dbl[])
        n105 = Divide(x="Grain 1 Orientation", y=w124) -> (x/y=w141:dbl[])
        n106 = Build Array(w142, w132, w141) -> (w140:T9)
        n107 = call "Matrix Transform Structure.vi"("Matrix Transform"=w140, "Original Structure"="Conventional Unit Cell") -> ("After Transform"=w130:T2)  [unwired: 9 in]
        n108 = case shown="\"Orthorhombic\", Default" "GB Geometric Type" {
          tunnel: [w152 w177 w187] -> w131
          tunnel: w130 -> [w151 w179 w188]
          frame "Orthorhombic", Default {
            w153 = -0.01 ("Z Min")
            n109 = Unbundle By Name("Grain 1 Size") -> ("Height"=w145:dbl, "Width"=w146:dbl, "Length"=w144:dbl, "Start"=w143:dbl)
            n110 = local read "Lattice Parameter"() -> (w148:dbl)
            n111 = Bundle("Z Min"=w153, "Width"=w146, "Z Min"=w153, "Height"=w145, "Start"=w143, "Length"=w144) -> (w150:T13)  [unwired: 1 in]
            n112 = Multiply(x=w150, y=w148) -> (x*y=w149:T13)
            n113 = call "Supercell Structure into a Box.vi"("Draw Box"=w149, "Subcrystal"=w151) -> ("Expanded cubic Structure"=w152:T2)  [unwired: 7 in, 2 out]
          }
          frame "Monoclinic" {
            w163 = 0.0 ("Z Min")
            w176 = -0.01 ("Z Min")
            n114 = local read "Lattice Parameter"() -> (w160:dbl)
            n115 = Unbundle By Name("Grain 1 Monoclinic size") -> ("Angle (deg)"=w157:dbl)
            n116 = Multiply(x="Grain 1 Monoclinic size", y=w160) -> (x*y=w159:T6)
            n117 = Divide(x=6.283185307179586, y=360.0) -> (x/y=w172:dbl)
            n118 = Multiply(x=w157, y=w172) -> (x*y=w171:dbl)
            n119 = Unbundle By Name(w159) -> ("Height"=w168:dbl, "Width"=w156:dbl, "Length"=w165:dbl, "Start"=w175:dbl)
            n120 = Sine & Cosine(0:w171) -> (1:w170:dbl, 2:w169:dbl)
            n121 = Multiply(x=w168, y=w169) -> (x*y=w167:dbl)
            n122 = Multiply(x=w168, y=w170) -> (x*y=w155:dbl)
            n123 = disable-structure shown="Enabled" {
              disable-tunnel: w156 -> [w182 _]
              disable-tunnel: w155 -> [w181 w183]
              disable-tunnel: [w180 w183] -> w154
              frame Disabled {
                n124 = Add(x=w182, y=w181) -> (x+y=w180:dbl)
              }
              frame Enabled {
              }
            }
            n125 = Bundle("Z Min"=w176, w154, "Z Min"=w176, w155, "Start"=w175, "Length"=w165) -> (w161:T14)  [unwired: 1 in]
            n126 = call "Supercell Structure into a Box.vi"("Draw Box"=w161, "Subcrystal"=w179) -> ("Expanded cubic Structure"=w178:T2)  [unwired: 7 in, 2 out]
            n127 = Build Array(w167, w155, w163) -> (w166:dbl[])
            n128 = Build Array(w154, w163, w163) -> (w162:dbl[])
            n129 = Build Array(w163, w163, w165) -> (w164:dbl[])
            n130 = call "Crop Supercell to new subcell.vi"("New Lattice Vector c"=w164, "New Lattice Vector b"=w166, "New Lattice Vector a"=w162, "Supercell Structure"=w178) -> ("Reduced Structure"=w177:T2)  [unwired: 7 in]
          }
          frame "Triclinic" {
            n131 = disable-structure shown="Enabled" {
              disable-tunnel: w188 -> [w205 w210]
              disable-tunnel: [w203 w206] -> w187
              disable-tunnel: "New Lattice Vector a" -> [w192 w208]
              disable-tunnel: "New Lattice Vector b" -> [w191 w209]
              disable-tunnel: "New Lattice Vector c" -> [w190 w207]
              frame Disabled {
                w197 = -0.01 ("Z Min")
                n132 = Compound Arithmetic op=ADD(w192, w191, w190) -> (w189:dbl[])
                n133 = Build Array(w192, w191, w190, w189) -> (w202:dbl[][])
                n134 = Index Array(array=w202, index (col) #1=0 ("disabled index (col)")) -> (element #1=w200:dbl[], element #2=w199:dbl[], element #3=w198:dbl[])  [unwired: 5 in]
                n135 = Array Max & Min(array=w200) -> (max value=w196:dbl)  [unwired: 3 out]
                n136 = Array Max & Min(array=w199) -> (max value=w195:dbl)  [unwired: 3 out]
                n137 = Array Max & Min(array=w198) -> (max value=w194:dbl)  [unwired: 3 out]
                n138 = Bundle("Z Min"=w197, w196, "Z Min"=w197, w195, "Z Min"=w197, w194) -> (w193:T15)  [unwired: 1 in]
                n139 = call "Supercell Structure into a Box.vi"("Draw Box"=w193, "Subcrystal"=w205) -> ("Expanded cubic Structure"=w204:T2)  [unwired: 7 in, 2 out]
                n140 = call "Crop Supercell to new subcell.vi"("New Lattice Vector c"=w190, "New Lattice Vector b"=w191, "New Lattice Vector a"=w192, "Supercell Structure"=w204) -> ("Reduced Structure"=w203:T2)  [unwired: 7 in]
              }
              frame Enabled {
                n141 = call "Grow primitive into new lattice vectors.vi"("New Lattice Vector c"=w207, "New Lattice Vector b"=w209, "New Lattice Vector a"=w208, "Primitive"=w210) -> ("Expanded to new Vectors"=w206:T2)  [unwired: 5 in, 2 out]
              }
            }
          }
        }
        "Grain 1" <- w131
        n142 = local read "Grain 1 Object"() -> (w135:refnum<vi>)
        n143 = Close Reference(reference=w135) -> (error out=w134:errorcluster)  [unwired: 1 in]
        n144 = call <vilib>:"Create Object.vi"("error in (no error)"=w134, "Name"="Base") -> ("Scene:New Object"=w138:refnum<vi>)  [unwired: 9 out]
        n145 = stacked-sequence {
          tunnel: w131 -> [_]
          frame #0 {
            n146 = property on="Make GB" class="Bool (strict)"("Val(Sgnl)"=TRUE ("Value (Signaling)")) -> ()  [unwired: 2 in, 2 out]
          }
        }
        n147 = call "Render Structure.vi"("Options"="Options", "Scale"="Zoom Scale", "Atomic Structure"=w131, "Base Object"=w138) -> ("Object with atoms"=w133:refnum<vi>)  [unwired: 7 in]
        "Grain 1 Render" <- w133
        n148 = local write "Grain 1 Object"(w133) -> ()
      }
      event "Add Tilt Angle": Value Change {
        n149 = event-data() -> ()  [unwired: 1 in, 5 out]
        n150 = local read "Mutual Viewing Angle"() -> (w212:dbl[])
        n151 = Greater Or Equal To 0?(x="Add Tilt Angle") -> (x >= 0?=w213:bool)
        n152 = case shown="False" w213 {
          tunnel: [w219 w221] -> w215
          tunnel: w212 -> [w220 w221]
          frame False {
            n153 = Negate(x=w220) -> (-x=w219:dbl[])
          }
          frame True {
          }
        }
        n154 = local read "Grain 1 Orientation"() -> (w217:dbl[])
        n155 = call "Make Rotation Matrix.vi"("Rotation Axis"=w215, "Rotation Angle (Degree)"="Add Tilt Angle") -> ("Rotation Matrix"=w218:T9)  [unwired: 9 in]
        n156 = call-poly <vilib>:"A x B.vi"("Matrix A"=w218, "Vector V'"=w217) -> ("V' x A"=w216:dbl[])  [unwired: 1 out]
        n157 = property on="Grain 2 Orientation" class="Arr (strict)"("Val(Sgnl)"=w216) -> ()  [unwired: 2 in, 2 out]
      }
      event "Make Grain 2": Value Change {
        n158 = event-data() -> ()  [unwired: 1 in, 5 out]
        n159 = local read "Mutual Viewing Angle"() -> (w232:dbl[])
        n160 = local read "Grain 1 Orientation"() -> (w228:dbl[])
        n161 = call "Angle between two vectors.vi"("Vector 2"="Grain 2 Orientation", "Vector 1"=w228) -> ("Angle (Degrees)"=w235:dbl)  [unwired: 7 in, 2 out]
        n162 = call-poly <vilib>:"Vector Norm.vi"("Input Vector"=w232) -> ("norm"=w250:dbl)  [unwired: 9 in, 1 out]
        n163 = call <vilib>:"Cross Product.vi"("B Vector"="Grain 2 Orientation", "A Vector"=w232) -> ("Cross Product"=w245:dbl[])  [unwired: 8 in, 1 out]
        n164 = call-poly <vilib>:"Vector Norm.vi"("Input Vector"="Grain 2 Orientation") -> ("norm"=w248:dbl)  [unwired: 9 in, 1 out]
        n165 = local write "Add Tilt Angle"(w235) -> ()
        n166 = Divide(x=w232, y=w250) -> (x/y=w247:dbl[])
        n167 = Divide(x="Grain 2 Orientation", y=w248) -> (x/y=w246:dbl[])
        n168 = call-poly <vilib>:"Vector Norm.vi"("Input Vector"=w245) -> ("norm"=w249:dbl)  [unwired: 9 in, 1 out]
        n169 = Divide(x=w245, y=w249) -> (x/y=w231:dbl[])
        n170 = Build Array(w247, w231, w246) -> (w229:T9)
        n171 = disable-structure shown="Enabled" {
          disable-tunnel: w229 -> [w316 _]
          disable-tunnel: w228 -> [w315 _]
          disable-tunnel: [w314 dbl[] [0.0, 0.0, 1.0] ("Rotation Axis")] -> w227
          disable-tunnel: "Grain 2 Orientation" -> [_ _]
          frame Disabled {
            n172 = call-poly <vilib>:"A x B.vi"("Vector"=w315, "A"=w316) -> ("A x Vector"=w314:dbl[])  [unwired: 1 out]
          }
          frame Enabled {
          }
        }
        n173 = local read "Conventional Unit Cell"() -> (w226:T2)
        n174 = call "Make Rotation Matrix.vi"("Rotation Axis"=w227, "Rotation Angle (Degree)"="Twist Angle") -> ("Rotation Matrix"=w230:T9)  [unwired: 9 in]
        n175 = local read "GB Geometric Type"() -> (w222:T4)
        n176 = call-poly <vilib>:"A x B.vi"("B"=w229, "A"=w230) -> ("A x B"=w236:T9)  [unwired: 1 out]
        n177 = call "Matrix Transform Structure.vi"("Matrix Transform"=w236, "Original Structure"=w226) -> ("After Transform"=w234:T2)  [unwired: 9 in]
        n178 = call "Translate Structure.vi"("Translation Vector (Cartesian)"="Translation Vector", "Atomic Structure"=w234) -> ("Shifted Structure"=w224:T2)  [unwired: 9 in]
        "Grain 2 Primative" <- w224
        n179 = case shown="\"Triclinic\"" w222 {
          tunnel: [w260 w284 w291] -> w223
          tunnel: w224 -> [w259 w286 w290]
          frame "Orthorhombic", Default {
            w261 = -0.01 ("Z Min")
            n180 = Unbundle By Name("Grain 2 Size") -> ("Height"=w254:dbl, "Width"=w255:dbl, "Length"=w253:dbl, "Start"=w252:dbl)
            n181 = local read "Lattice Parameter"() -> (w256:dbl)
            n182 = Bundle("Z Min"=w261, "Width"=w255, "Z Min"=w261, "Height"=w254, "Start"=w252, "Length"=w253) -> (w258:T13)  [unwired: 1 in]
            n183 = Multiply(x=w258, y=w256) -> (x*y=w257:T13)
            n184 = call "Supercell Structure into a Box.vi"("Draw Box"=w257, "Subcrystal"=w259) -> ("Expanded cubic Structure"=w260:T2)  [unwired: 7 in, 2 out]
          }
          frame "Monoclinic" {
            w269 = 0.0 ("Z Min")
            w283 = -0.01 ("Z Min")
            n185 = local read "Lattice Parameter"() -> (w266:dbl)
            n186 = Multiply(x="Grain 2 Monoclinic size", y=w266) -> (x*y=w265:T6)
            n187 = Unbundle By Name(w265) -> ("Height"=w274:dbl, "Width"=w267:dbl, "Length"=w271:dbl, "Start"=w282:dbl)
            n188 = Unbundle By Name("Grain 2 Monoclinic size") -> ("Angle (deg)"=w263:dbl)
            n189 = Divide(x=6.283185307179586, y=360.0) -> (x/y=w279:dbl)
            n190 = Multiply(x=w263, y=w279) -> (x*y=w278:dbl)
            n191 = Sine & Cosine(0:w278) -> (1:w277:dbl, 2:w275:dbl)
            n192 = Multiply(x=w274, y=w275) -> (x*y=w273:dbl)
            n193 = Multiply(x=w274, y=w277) -> (x*y=w276:dbl)
            n194 = Bundle("Z Min"=w283, "Width"=w267, "Z Min"=w283, w276, "Start"=w282, "Length"=w271) -> (w262:T16)  [unwired: 1 in]
            n195 = call "Supercell Structure into a Box.vi"("Draw Box"=w262, "Subcrystal"=w286) -> ("Expanded cubic Structure"=w285:T2)  [unwired: 7 in, 2 out]
            n196 = Build Array(w273, w276, w269) -> (w272:dbl[])
            n197 = Build Array(w267, w269, w269) -> (w268:dbl[])
            n198 = Build Array(w269, w269, w271) -> (w270:dbl[])
            n199 = call "Crop Supercell to new subcell.vi"("New Lattice Vector c"=w270, "New Lattice Vector b"=w272, "New Lattice Vector a"=w268, "Supercell Structure"=w285) -> ("Reduced Structure"=w284:T2)  [unwired: 7 in]
          }
          frame "Triclinic" {
            n200 = disable-structure shown="Enabled" {
              disable-tunnel: [w296 w309] -> w291
              disable-tunnel: w290 -> [w295 w312]
              disable-tunnel: "New Lattice Vector a 2" -> [w294 w313]
              disable-tunnel: "New Lattice Vector b 2" -> [w293 w311]
              disable-tunnel: "New Lattice Vector c 2" -> [w292 w310]
              frame Disabled {
                w302 = -0.01 ("Z Min")
                n201 = Compound Arithmetic op=ADD(w294, w293, w292) -> (w297:dbl[])
                n202 = Build Array(w294, w293, w292, w297) -> (w307:dbl[][])
                n203 = Index Array(array=w307, index (col) #1=0 ("disabled index (col)")) -> (element #1=w305:dbl[], element #2=w304:dbl[], element #3=w303:dbl[])  [unwired: 5 in]
                n204 = Array Max & Min(array=w305) -> (max value=w301:dbl)  [unwired: 3 out]
                n205 = Array Max & Min(array=w304) -> (max value=w300:dbl)  [unwired: 3 out]
                n206 = Array Max & Min(array=w303) -> (max value=w299:dbl)  [unwired: 3 out]
                n207 = Bundle("Z Min"=w302, w301, "Z Min"=w302, w300, "Z Min"=w302, w299) -> (w298:T15)  [unwired: 1 in]
                n208 = call "Supercell Structure into a Box.vi"("Draw Box"=w298, "Subcrystal"=w295) -> ("Expanded cubic Structure"=w308:T2)  [unwired: 7 in, 2 out]
                n209 = call "Crop Supercell to new subcell.vi"("New Lattice Vector c"=w292, "New Lattice Vector b"=w293, "New Lattice Vector a"=w294, "Supercell Structure"=w308) -> ("Reduced Structure"=w296:T2)  [unwired: 7 in]
              }
              frame Enabled {
                n210 = call "Grow primitive into new lattice vectors.vi"("New Lattice Vector c"=w310, "New Lattice Vector b"=w311, "New Lattice Vector a"=w313, "Primitive"=w312) -> ("Expanded to new Vectors"=w309:T2)  [unwired: 5 in, 2 out]
              }
            }
          }
        }
        "Grain 2" <- w223
        n211 = local read "Grain 2 Object"() -> (w239:refnum<vi>)
        n212 = local read "Zoom Scale"() -> (w242:dbl)
        n213 = local read "Options"() -> (w241:cluster{"Border?":bool, "Bonds?":bool})
        n214 = stacked-sequence {
          tunnel: w223 -> [_]
          frame #0 {
            n215 = property on="Make GB" class="Bool (strict)"("Val(Sgnl)"=TRUE ("Value (Signaling)")) -> ()  [unwired: 2 in, 2 out]
          }
        }
        n216 = Close Reference(reference=w239) -> (error out=w238:errorcluster)  [unwired: 1 in]
        n217 = call <vilib>:"Create Object.vi"("error in (no error)"=w238, "Name"="Base") -> ("Scene:New Object"=w243:refnum<vi>)  [unwired: 9 out]
        n218 = call "Render Structure.vi"("Options"=w241, "Scale"=w242, "Atomic Structure"=w223, "Base Object"=w243) -> ("Object with atoms"=w240:refnum<vi>)  [unwired: 7 in]
        "Grain 2 Render" <- w240
        n219 = local write "Grain 2 Object"(w240) -> ()
      }
      event "Make GB": Value Change {
        n220 = event-data() -> ()  [unwired: 1 in, 5 out]
        n221 = local read "Grain Boundary Object"() -> (w330:refnum<vi>)
        n222 = local read "Grain 1"() -> (w332:T2)
        n223 = Unbundle By Name(w332) -> ("Lattice vector c"=w327:dbl[])
        n224 = local read "Grain 2"() -> (w337:T2)
        n225 = Close Reference(reference=w330) -> (error out=w329:errorcluster)  [unwired: 1 in]
        n226 = disable-structure shown="Enabled" {
          disable-tunnel: w337 -> [w341 w343]
          disable-tunnel: w332 -> [w340 w344]
          disable-tunnel: [w339 w342] -> w328
          disable-tunnel: w327 -> [w338 _]
          frame Disabled {
            n227 = call "Merge Two Structures (Cuboid).vi"("Translation Vector (1 to 2)"=w338, "Atomic Structure 2"=w341, "Atomic Structure 1"=w340) -> ("Atomic Structure of 1 + 2 by T"=w339:T2)  [unwired: 8 in]
          }
          frame Enabled {
            n228 = call "Merge two co-incident cells.vi"("Grain 2"=w343, "Grain 1"=w344) -> ("Joined GB"=w342:T2)  [unwired: 9 in]
          }
        }
        n229 = call <vilib>:"Create Object.vi"("error in (no error)"=w329, "Name"="Base") -> ("Scene:New Object"=w335:refnum<vi>)  [unwired: 9 out]
        n230 = local read "Grain 1 Orientation"() -> (w324:dbl[])
        n231 = local read "Grain 2 Orientation"() -> (w323:dbl[])
        n232 = local read "Translation Vector"() -> (w321:dbl[])
        n233 = local read "Zoom Scale"() -> (w334:dbl)
        n234 = local read "Twist Angle"() -> (w322:dbl)
        n235 = local read "Options"() -> (w333:cluster{"Border?":bool, "Bonds?":bool})
        n236 = call "Render Structure.vi"("Options"=w333, "Scale"=w334, "Atomic Structure"=w328, "Base Object"=w335) -> ("Object with atoms"=w331:refnum<vi>)  [unwired: 7 in]
        "Grain Boundary Render" <- w331
        n237 = Bundle("Grain 1 Orientation"=w324, "Grain 2 Orientation"=w323, "Twist Angle"=w322, "Translation Vector"=w321) -> (→"Grain Boundary Definition":T12)  [unwired: 1 in]
        n238 = local write "Grain Boundary Object"(w331) -> ()
        n239 = local write "Timeout Activity"("Analyze GB" ("Timeout Activity")) -> ()
        n240 = Bundle By Name(cluster=w328, "Structure Name"="Grain Boundary") -> (→"Grain Boundary":T2)
      }
      event "Crop to Smallest Repeating": Value Change {
        n241 = event-data() -> ()  [unwired: 1 in, 5 out]
        n242 = local read "Grain Boundary"() -> (w346:T2)
        n243 = case shown="False" "Force Orthorhombic?" {
          tunnel: [w359 w378] -> w351
          tunnel: "Slab X" -> [w362 w377]
          tunnel: "Slab Y" -> [w361 w376]
          tunnel: "Tolerance (A)" -> [w360 w375]
          tunnel: w346 -> [w363 w374]
          frame False {
            n244 = Unbundle By Name(w363) -> ("Lattice vector c"=w365:dbl[])
            n245 = call "Find Repeating Monoclinic GB.vi"("Tolerance (A)"=w360, "Slab Y"=w361, "Slab X"=w362, "Supercell Structure"=w363) -> ("New Lattice Vector b"=w368:dbl[], "New Lattice Vector a"=w367:dbl[])  [unwired: 5 in, 1 out]
            n246 = Multiply(x=w365, y=1.0) -> (x*y=w364:dbl[])
            n247 = call "Crop Supercell to new subcell.vi"("New Lattice Vector c"=w364, "New Lattice Vector b"=w368, "New Lattice Vector a"=w367, "Supercell Structure"=w363) -> ("Reduced Structure"=w359:T2)  [unwired: 7 in]
          }
          frame True {
            n248 = call "Find Repeating Ortho-Subset in GB.vi"("Tolerance (A)"=w375, "Slab Y"=w376, "Slab X"=w377, "Grain Boundary"=w374) -> ("Repeating Y Length Scale"=w370:dbl, "Subset Y found?!"=w369:bool, "Repeating X Length Scale"=w372:dbl, "Subset X found?!"=w371:bool)  [unwired: 4 in]
            "Repeating X Length Scale" <- w372
            "Subset for X?" <- w371
            "Repeating Y Length Scale" <- w370
            "Subset for Y?" <- w369
            n249 = case shown="True" w371 {
              tunnel: w374 -> [w385 w390]
              tunnel: [w385 w387] -> w373
              tunnel: w372 -> [_ w386]
              frame False {
              }
              frame True {
                n250 = call "Crop Structure.vi"("Cropping Index"=enum16{"X", "Y", "Z"}."X", "Upper Bound Z"=w386, "Lower bound Z"=0.0, "Input Structure"=w390) -> ("Cropped Structure"=w387:T2)  [unwired: 7 in]
              }
            }
            n251 = case shown="True" w369 {
              tunnel: w373 -> [w379 w384]
              tunnel: w370 -> [_ w382]
              tunnel: [w379 w380] -> w378
              frame False {
              }
              frame True {
                n252 = call "Crop Structure.vi"("Cropping Index"=enum16{"X", "Y", "Z"}."Y", "Upper Bound Z"=w382, "Lower bound Z"=0.0, "Input Structure"=w384) -> ("Cropped Structure"=w380:T2)  [unwired: 7 in]
              }
            }
          }
        }
        n253 = local read "Zoom Scale"() -> (w355:dbl)
        n254 = local read "Grain Boundary Object"() -> (w354:refnum<vi>)
        n255 = Unbundle By Name(w351) -> ("# of atoms"=w350:i32)
        n256 = local write "Grain Boundary"(w351) -> ()
        n257 = local read "Options"() -> (w356:cluster{"Border?":bool, "Bonds?":bool})
        n258 = local write "# of Atoms"(w350) -> ()
        n259 = Close Reference(reference=w354) -> (error out=w352:errorcluster)  [unwired: 1 in]
        n260 = call <vilib>:"Create Object.vi"("error in (no error)"=w352, "Name"="Base") -> ("Scene:New Object"=w357:refnum<vi>)  [unwired: 9 out]
        n261 = call "Render Structure.vi"("Options"=w356, "Scale"=w355, "Atomic Structure"=w351, "Base Object"=w357) -> ("Object with atoms"=w353:refnum<vi>)  [unwired: 7 in]
        n262 = local write "Grain Boundary Object"(w353) -> ()
        n263 = local write "Grain Boundary Render"(w353) -> ()
      }
      event "Remove Close Atoms": Value Change {
        n264 = event-data() -> ()  [unwired: 1 in, 5 out]
        n265 = local read "Grain 1 Size"() -> (w392:T5)
        n266 = Unbundle By Name(w392) -> ("Length"=w391:dbl)
        n267 = local read "Grain Boundary"() -> (w398:T2)
        n268 = call "Remove Close Atoms on GB.vi"("Grain Boundary Location (A)"=w391, "Edge Duplication Range"=3.0, "Minimally Allowable Distance (A)"="Minimally Allowable Distance (A)", "Structure"=w398) -> ("# of Atoms Removed"=→"# of Atoms Removed":i32, "Structure with atoms removed"=w396:T2)  [unwired: 6 in]
        n269 = local read "Grain Boundary Object"() -> (w401:refnum<vi>)
        n270 = local read "Zoom Scale"() -> (w402:dbl)
        n271 = local write "Grain Boundary"(w396) -> ()
        n272 = local read "Options"() -> (w403:cluster{"Border?":bool, "Bonds?":bool})
        n273 = Close Reference(reference=w401) -> (error out=w399:errorcluster)  [unwired: 1 in]
        n274 = call <vilib>:"Create Object.vi"("error in (no error)"=w399, "Name"="Base") -> ("Scene:New Object"=w397:refnum<vi>)  [unwired: 9 out]
        n275 = call "Render Structure.vi"("Options"=w403, "Scale"=w402, "Atomic Structure"=w396, "Base Object"=w397) -> ("Object with atoms"=w400:refnum<vi>)  [unwired: 7 in]
        n276 = local write "Grain Boundary Object"(w400) -> ()
        n277 = local write "Grain Boundary Render"(w400) -> ()
      }
      event "Save to POSCAR": Value Change {
        n278 = event-data() -> ()  [unwired: 1 in, 5 out]
        n279 = call "Save to POSCAR"() -> ("selected path"=w408:path)  [unwired: 12 in, 3 out]
        n280 = Build Path(base path=w408, name or relative path="Structure Name") -> (appended path=w406:path)
        n281 = Create Folder(path (use dialog)=w406) -> (created path=w405:path)  [unwired: 2 in, 2 out]
        n282 = stacked-sequence {
          tunnel: "Structure Name" -> [w410 _]
          tunnel: w405 -> [w409 w451]
          frame #0 {
            n283 = local read "Grain Boundary"() -> (w415:T2)
            n284 = Build Path(base path=w409, name or relative path="POSCAR") -> (appended path=w412:path)
            n285 = Bundle By Name(cluster=w415, "Structure Name"=w410) -> (w414:T2)
            n286 = call "Atoms to POSCAR.vi"("Atomic Structure"=w414) -> ("POSCAR File"=w411:string)  [unwired: 10 in]
            n287 = Write to Text File(file (use dialog)=w412, text=w411) -> ()  [unwired: 2 in, 3 out]
          }
          frame #1 {
            w426 = "," ("string")
            w423 = i16 2 ("precision (6)")
            w442 = "," ("string")
            w445 = "," ("string")
            n288 = local read "Grain 1 Orientation"() -> (w435:dbl[])
            n289 = local read "Grain 2 Orientation"() -> (w437:dbl[])
            n290 = local read "Translation Vector"() -> (w424:dbl[])
            n291 = local read "Grain 1 Size"() -> (w417:T5)
            n292 = Build Path(base path=w451, name or relative path="README.txt") -> (appended path=w453:path)
            n293 = Unbundle By Name(w417) -> ("Start"=w416:dbl)  [unwired: 3 out]
            n294 = Number To Fractional String(number=w435, precision (6)=w423) -> (F-format string=w434:string[])  [unwired: 2 in]
            n295 = Number To Fractional String(number=w437, precision (6)=w423) -> (F-format string=w436:string[])  [unwired: 2 in]
            n296 = Number To Fractional String(number=w424, precision (6)=w423) -> (F-format string=w429:string[])  [unwired: 2 in]
            n297 = local read "Overlap Region"() -> (w421:dbl)
            n298 = local read "Add Tilt Angle"() -> (w439:dbl)
            n299 = Index Array(array=w434) -> (element #1=w447:string, element #2=w446:string, element #3=w444:string)  [unwired: 3 in]
            n300 = Index Array(array=w436) -> (element #1=w440:string, element #2=w441:string, element #3=w443:string)  [unwired: 3 in]
            n301 = Index Array(array=w429) -> (element #1=w428:string, element #2=w427:string, element #3=w425:string)  [unwired: 3 in]
            n302 = local read "Twist Angle"() -> (w438:dbl)
            n303 = Concatenate Strings(w447, w445, w446, w445, w444) -> (w433:string)
            n304 = Concatenate Strings(w440, w442, w441, w442, w443) -> (w432:string)
            n305 = Number To Fractional String(number=w438) -> (F-format string=w431:string)  [unwired: 3 in]
            n306 = Number To Fractional String(number=w439) -> (F-format string=w430:string)  [unwired: 3 in]
            n307 = Concatenate Strings(w428, w426, w427, w426, w425) -> (w422:string)
            n308 = Number To Fractional String(number=w421) -> (F-format string=w420:string)  [unwired: 3 in]
            n309 = Number To Fractional String(number=w416) -> (F-format string=w419:string)  [unwired: 3 in]
            n310 = Build Array(w433, w432, w431, w430, w422, w420, w419) -> (w418:string[])
            n311 = Build Array(string[] ["Grain 1 Orientation", "Grain 2 Orientation", "Twist Angle (Degree)", "Tilt Angle (Degree)", "Translation (x,y,z)", "Overlap Length (A)", "Grain 1 Start (A)"], w418) -> (w449:string[][])
            n312 = Transpose 2D Array(2D array=w449) -> (transposed array=w448:string[][])
            n313 = call-poly <vilib>:"Write To Spreadsheet File.vi"("2D data"=w448, "file path (dialog if empty)"=w453) -> ()  [unwired: 6 in, 1 out]
          }
        }
      }
      event "Save into GULP": Value Change {
        w465 = "," ("string")
        w462 = i16 2 ("precision (6)")
        w481 = "," ("string")
        w484 = "," ("string")
        n314 = event-data() -> ()  [unwired: 1 in, 5 out]
        n315 = local read "Grain 1 Size"() -> (w455:T5)
        n316 = local read "Grain 1 Orientation"() -> (w474:dbl[])
        n317 = local read "Grain 2 Orientation"() -> (w476:dbl[])
        n318 = local read "Translation Vector"() -> (w463:dbl[])
        n319 = Unbundle By Name(w455) -> ("Start"=w454:dbl)  [unwired: 3 out]
        n320 = Number To Fractional String(number=w474, precision (6)=w462) -> (F-format string=w473:string[])  [unwired: 2 in]
        n321 = Number To Fractional String(number=w476, precision (6)=w462) -> (F-format string=w475:string[])  [unwired: 2 in]
        n322 = Number To Fractional String(number=w463, precision (6)=w462) -> (F-format string=w468:string[])  [unwired: 2 in]
        n323 = local read "Overlap Region"() -> (w460:dbl)
        n324 = local read "Add Tilt Angle"() -> (w478:dbl)
        n325 = Index Array(array=w473) -> (element #1=w486:string, element #2=w485:string, element #3=w483:string)  [unwired: 3 in]
        n326 = Index Array(array=w475) -> (element #1=w479:string, element #2=w480:string, element #3=w482:string)  [unwired: 3 in]
        n327 = Index Array(array=w468) -> (element #1=w467:string, element #2=w466:string, element #3=w464:string)  [unwired: 3 in]
        n328 = local read "Twist Angle"() -> (w477:dbl)
        n329 = Concatenate Strings(w486, w484, w485, w484, w483) -> (w472:string)
        n330 = Concatenate Strings(w479, w481, w480, w481, w482) -> (w471:string)
        n331 = Number To Fractional String(number=w477) -> (F-format string=w470:string)  [unwired: 3 in]
        n332 = Number To Fractional String(number=w478) -> (F-format string=w469:string)  [unwired: 3 in]
        n333 = Concatenate Strings(w467, w465, w466, w465, w464) -> (w461:string)
        n334 = Number To Fractional String(number=w460) -> (F-format string=w459:string)  [unwired: 3 in]
        n335 = Number To Fractional String(number=w454) -> (F-format string=w458:string)  [unwired: 3 in]
        n336 = local read "Structure Name"() -> (w492:string)
        n337 = Build Array(w472, w471, w470, w469, w461, w459, w458) -> (w457:string[])
        n338 = Build Array(string[] ["Grain 1 Orientation", "Grain 2 Orientation", "Twist Angle (Degree)", "Tilt Angle (Degree)", "Translation (x,y,z)", "Overlap Length (A)", "Grain 1 Start (A)"], w457) -> (w487:string[][])
        n339 = call <vilib>:"Search and Replace Pattern.vi"("string"=w492, "regular expression (\"\")"="[\\s()\\[\\]]" ("regular expression (\"\")"), "replace string (\"\")"="_" ("replace string (\"\")"), "replace all? (F)"=TRUE) -> ("result string"=w491:string)  [unwired: 1 in, 1 out]
        n340 = Transpose 2D Array(2D array=w487) -> (transposed array=w489:string[][])
        n341 = local read "Grain Boundary"() -> (w502:T2)
        n342 = call "Save to GULP"() -> ("selected path"=w499:path)  [unwired: 12 in, 3 out]
        n343 = Array To Spreadsheet String(array=w489, 3:"%s" ("format string")) -> (spreadsheet string=w456:string)  [unwired: 1 in]
        n344 = Concatenate Strings(w491, ".gin" ("string")) -> (w497:string)
        n345 = Build Path(base path=w499, name or relative path=w497) -> (appended path=w496:path)
        n346 = call "Atoms to GULP File.vi"("Title and Comments"=w456, "Relaxation Type"="Relaxation Type", "Structure"=w502) -> ("GULP File"=w500:string)  [unwired: 8 in]
        n347 = Write to Text File(file (use dialog)=w496, text=w500) -> ()  [unwired: 2 in, 3 out]
      }
      event "Save to GB config file": Value Change {
        n348 = event-data() -> ()  [unwired: 1 in, 5 out]
        n349 = local read "Grain Boundary Definition"() -> (w522:T1)
        n350 = local read "Grain 2 Size"() -> (w521:T5)
        n351 = local read "Grain 1 Size"() -> (w520:T5)
        n352 = local read "Structure Name"() -> (w507:string)
        n353 = Cluster To Array(cluster=w520) -> (array=w515:dbl[])
        n354 = Cluster To Array(cluster=w521) -> (array=w514:dbl[])
        n355 = Unbundle(w522) -> ("Grain 1 Orientation"=w519:dbl[], "Grain 2 Orientation"=w518:dbl[], "Twist Angle (Deg)"=w517:dbl, "Translation Vector"=w516:dbl[])
        n356 = Build Array (concatenate)(w519, w518, w517, w516, w515, w514) -> (w513:dbl[])
        n357 = Concatenate Strings(w507, ".GB" ("string")) -> (w511:string)
        n358 = Number To Fractional String(number=w513) -> (F-format string=w508:string[])  [unwired: 3 in]
        n359 = call "File Dialog"("default name"=w511, "pattern (all files)"="*.GB") -> ("selected path"=w509:path)  [unwired: 10 in, 3 out]
        n360 = Build Array (concatenate)(w507, w508) -> (w506:string[])
        n361 = Build Array(string[] ["Name", "Grain 1, h", "Grain 1, k", "Grain 1, l", "Grain 2, h", "Grain 2, k", "Grain 2, l", "Twist Angle (Degree)", "Translation x", "Translation y", "Translation z", "Grain 1, Height", "Grain 1, Width", "Grain 1, Length", "Grain 1, Start", "Grain 2, Height", "Grain 2, Width", "Grain 2, Length", "Grain 2, Start"], w506) -> (w505:string[][])
        n362 = Transpose 2D Array(2D array=w505) -> (transposed array=w504:string[][])
        n363 = call-poly <vilib>:"Write To Spreadsheet File.vi"("2D data"=w504, "file path (dialog if empty)"=w509) -> ()  [unwired: 6 in, 1 out]
      }
      event "Load GB Config": Value Change {
        n364 = event-data() -> ()  [unwired: 1 in, 5 out]
        n365 = call "Load GB"("pattern (all files)"="*.GB") -> ("selected path"=w524:path)  [unwired: 11 in, 3 out]
        n366 = call-poly <vilib>:"Read From Spreadsheet File.vi"("file path (dialog if empty)"=w524) -> ("all rows"=w527:string[][])  [unwired: 6 in, 4 out]
        n367 = Index Array(array=w527, index (col)=1 ("disabled index (col)")) -> (element=w525:string[])  [unwired: 1 in]
        n368 = flat-sequence {
          tunnel: w525 -> [w552]
          frame #0 {
            n369 = Fract/Exp String To Number(string=w552) -> (number=w551:dbl[])  [unwired: 3 in, 1 out]
            n370 = Index Array(array=w551) -> (element #2=w550:dbl, element #3=w549:dbl, element #4=w548:dbl, element #5=w547:dbl, element #6=w546:dbl, element #7=w545:dbl, element #8=w543:dbl, element #9=w542:dbl, element #10=w541:dbl, element #11=w540:dbl, element #12=w538:dbl, element #13=w537:dbl, element #14=w536:dbl, element #15=w535:dbl, element #16=w533:dbl, element #17=w532:dbl, element #18=w531:dbl, element #19=w530:dbl)  [unwired: 19 in, 1 out]
            n371 = local write "Twist Angle"(w543) -> ()
            n372 = Build Array(w550, w549, w548) -> (w528:dbl[])
            n373 = Build Array(w547, w546, w545) -> (w544:dbl[])
            n374 = Build Array(w542, w541, w540) -> (w539:dbl[])
            n375 = Bundle("String"=w538, "String"=w537, "String"=w536, "String"=w535) -> (w534:T17)  [unwired: 1 in]
            n376 = Bundle("String"=w533, "String"=w532, "String"=w531, "String"=w530) -> (w529:T17)  [unwired: 1 in]
            n377 = local write "Translation Vector"(w539) -> ()
            n378 = local write "Grain 1 Orientation"(w528) -> ()
            n379 = local write "Grain 2 Orientation"(w544) -> ()
            n380 = local write "Grain 1 Size"(w534) -> ()
            n381 = local write "Grain 2 Size"(w529) -> ()
          }
          frame #1 {
            n382 = property on="Make Grain 1" class="Bool (strict)"("Val(Sgnl)"=TRUE ("Value (Signaling)")) -> (error out=w555:errorcluster)  [unwired: 2 in, 1 out]
            n383 = property on="Make Grain 2" class="Bool (strict)"(error in=w555, "Val(Sgnl)"=TRUE ("Value (Signaling)")) -> ()  [unwired: 1 in, 2 out]
          }
        }
      }
      event "Suggest Sizes": Value Change {
        n384 = event-data() -> ()  [unwired: 1 in, 5 out]
        n385 = local read "Grain 1 Orientation"() -> (w562:dbl[])
        n386 = local read "Grain 2 Orientation"() -> (w561:dbl[])
        n387 = local read "Mutual Viewing Angle"() -> (w558:dbl[])
        n388 = local read "Twist Angle"() -> (w560:dbl)
        n389 = local read "GB Geometric Type"() -> (w556:T4)
        n390 = Bundle("Grain 1 Orientation"=w562, "Grain 2 Orientation"=w561, "Twist Angle"=w560) -> (w559:T18)  [unwired: 1 in]
        n391 = case shown="\"Orthorhombic\", Default" w556 {
          tunnel: w559 -> [w571 w640]
          tunnel: w558 -> [w569 _]
          tunnel: "Integer Tolerance" -> [w570 w639]
          frame "Orthorhombic", Default {
            w580 = -0.001 ("y")
            n392 = call "Predict Cuboid GB Dimensions.vi"("Mutual Viewing Angle"=w569, "Tolerance"=w570, "Grain Boundary Macro Definition"=w571) -> ("Suggested Cuboid Dimensions (proportional)"=w573:T19)  [unwired: 6 in, 2 out]
            n393 = Cluster To Array(cluster=w573) -> (array=w584:dbl[])
            n394 = Subtract(x=w573, y=0.001) -> (x-y=w581:T19)
            n395 = Unbundle By Name(w581) -> ("Grain 1 Length (prop)"=w568:dbl, "Grain 2 Length (prop)"=w567:dbl, "Grain 1 Height (prop)"=w565:dbl, "Grain 2 Height (prop)"=w578:dbl, "Grain 1 Width (prop)"=w564:dbl, "Grain 2 Width (prop)"=w579:dbl)
            n396 = Greater?(x=w584, y=10) -> (0:w585:bool[])
            n397 = Add(x=w568, y=w567) -> (x+y=w566:dbl)
            n398 = Or Array Elements(Boolean array=w585) -> (logical OR=w586:bool)
            n399 = Compound Arithmetic op=MULTIPLY(w566, w565, w564) -> (w563:dbl)
            n400 = Multiply(x=w563, y=0.0276277) -> (x*y=w572:dbl)
            n401 = Bundle("Grain 1 Height (prop)"=w565, "Grain 1 Width (prop)"=w564, "Grain 1 Length (prop)"=w568, "y"=w580) -> (w576:T20)  [unwired: 1 in]
            n402 = Bundle("Grain 2 Height (prop)"=w578, "Grain 2 Width (prop)"=w579, "Grain 2 Length (prop)"=w567, "y"=w580) -> (w575:T21)  [unwired: 1 in]
            n403 = case shown="True" w586 {
              tunnel: w572 -> [_ w595]
              tunnel: [w589 w593] -> w583
              tunnel: [w588 w592] -> w582
              tunnel: w576 -> [w589 w591]
              tunnel: w575 -> [w588 w590]
              frame False {
              }
              frame True {
                n404 = Number To Decimal String(number=w595) -> (decimal integer string=w594:string)  [unwired: 1 in]
                n405 = Concatenate Strings("This interface will be huge!\n\nProbably like " ("message"), w594, " atoms.\n\nAre you sure you want to create it?" ("string")) -> (w598:string)
                n406 = Two Button Dialog(message=w598, 1:"Limit to 20x" ("F button name (\"Cancel\")"), 2:"I know what I'm doing" ("T button name (\"OK\")")) -> (T button?=w601:bool)
                n407 = case shown="False" w601 {
                  tunnel: [w604 w619] -> w593
                  tunnel: [w602 w618] -> w592
                  tunnel: w591 -> [w609 w619]
                  tunnel: w590 -> [w607 w618]
                  frame False {
                    n408 = Cluster To Array(cluster=w609) -> (array=w608:dbl[])
                    n409 = Cluster To Array(cluster=w607) -> (array=w606:dbl[])
                    n410 = for {
                      tunnel: w608 -> [w616] mode=indexing
                      tunnel: [w614] -> w605 mode=indexing
                      w615 = 20.0 ("y")
                      n411 = Less?(x=w616, y=w615) -> (x < y?=w617:bool)
                      n412 = Select(t=w616, s=w617, f=w615) -> (s? t:f=w614:dbl)
                    }
                    n413 = for {
                      tunnel: w606 -> [w612] mode=indexing
                      tunnel: [w610] -> w603 mode=indexing
                      w611 = 20.0 ("y")
                      n414 = Less?(x=w612, y=w611) -> (x < y?=w613:bool)
                      n415 = Select(t=w612, s=w613, f=w611) -> (s? t:f=w610:dbl)
                    }
                    n416 = Array To Cluster(array=w605) -> (cluster=w604:T22)
                    n417 = Array To Cluster(array=w603) -> (cluster=w602:T22)
                  }
                  frame True {
                  }
                }
              }
            }
            n418 = property on="Grain 1 Size" class="Clust (strict)"("Val(Sgnl)"=w583) -> ()  [unwired: 2 in, 2 out]
            n419 = property on="Grain 2 Size" class="Clust (strict)"("Val(Sgnl)"=w582) -> ()  [unwired: 2 in, 2 out]
          }
          frame "Monoclinic" {
            n420 = call "Predict GB via Paralleogram.vi"("Tolerance"=w639, "Grain Boundary Macro Definition"=w640) -> ("Grain 2 Monoclinic size"=w637:T6, "Grain 1 Monoclinic size"=w638:T6)  [unwired: 8 in]
            n421 = local read "Lattice Parameter"() -> (w620:dbl)
            n422 = Unbundle By Name(w637) -> ("Length"=w635:dbl, "Width"=w633:dbl, "Height"=w632:dbl, "Angle (deg)"=w629:dbl)
            n423 = Unbundle By Name(w638) -> ("Length"=w636:dbl)
            n424 = Divide(x=6.283185307179586, y=360.0) -> (x/y=w628:dbl)
            n425 = Add(x=w636, y=w635) -> (x+y=w634:dbl)
            n426 = Multiply(x=w629, y=w628) -> (x*y=w627:dbl)
            n427 = Sine(x=w627) -> (sin(x)=w626:dbl)
            n428 = Compound Arithmetic op=MULTIPLY(w634, w633, w632, w626, w620, w620, w620) -> (w624:dbl)
            n429 = Multiply(x=w624, y=0.0276277) -> (x*y=w623:dbl)
            n430 = Greater?(x=w623, y=1500) -> (0:w622:bool)
            n431 = case shown="True" w622 {
              tunnel: [w644 w649] -> w641
              tunnel: [w643 w648] -> w621
              tunnel: w638 -> [w644 w647]
              tunnel: w637 -> [w643 w646]
              tunnel: w623 -> [_ w645]
              frame False {
              }
              frame True {
                n432 = Number To Decimal String(number=w645) -> (decimal integer string=w650:string)  [unwired: 1 in]
                n433 = Concatenate Strings("This interface will be huge!\n\nProbably like " ("message"), w650, " atoms.\n\nAre you sure you want to create it?" ("string")) -> (w653:string)
                n434 = Two Button Dialog(message=w653, 1:"Limit to 20x" ("F button name (\"Cancel\")"), 2:"I know what I'm doing" ("T button name (\"OK\")")) -> (T button?=w656:bool)
                n435 = case shown="False" w656 {
                  tunnel: [w657 w682] -> w649
                  tunnel: [w658 w681] -> w648
                  tunnel: w647 -> [w664 w682]
                  tunnel: w646 -> [w662 w681]
                  frame False {
                    n436 = Cluster To Array(cluster=w664) -> (array=w663:dbl[])
                    n437 = Cluster To Array(cluster=w662) -> (array=w661:dbl[])
                    n438 = for {
                      tunnel: w661 -> [w667] mode=indexing
                      tunnel: [w666] -> w659 mode=indexing
                      i -> [w665]
                      n439 = case shown="2" w665 {
                        tunnel: w667 -> [w668 w671]
                        tunnel: [w668 w669] -> w666
                        frame 2 {
                        }
                        frame Default {
                          w670 = 20.0 ("y")
                          n440 = Less?(x=w671, y=w670) -> (x < y?=w672:bool)
                          n441 = Select(t=w671, s=w672, f=w670) -> (s? t:f=w669:dbl)
                        }
                      }
                    }
                    n442 = for {
                      tunnel: w663 -> [w675] mode=indexing
                      tunnel: [w674] -> w660 mode=indexing
                      i -> [w673]
                      n443 = case shown="2" w673 {
                        tunnel: w675 -> [w676 w679]
                        tunnel: [w676 w677] -> w674
                        frame 2 {
                        }
                        frame Default {
                          w678 = 20.0 ("y")
                          n444 = Less?(x=w679, y=w678) -> (x < y?=w680:bool)
                          n445 = Select(t=w679, s=w680, f=w678) -> (s? t:f=w677:dbl)
                        }
                      }
                    }
                    n446 = Array To Cluster(array=w660) -> (cluster=w657:T23)
                    n447 = Array To Cluster(array=w659) -> (cluster=w658:T23)
                  }
                  frame True {
                  }
                }
              }
            }
            n448 = property on="Grain 1 Monoclinic size" class="Clust (strict)"("Val(Sgnl)"=w641) -> ()  [unwired: 2 in, 2 out]
            n449 = property on="Grain 2 Monoclinic size" class="Clust (strict)"("Val(Sgnl)"=w621) -> ()  [unwired: 2 in, 2 out]
          }
        }
      }
      event "Load G1 VESTA": Value Change {
        n450 = event-data() -> ()  [unwired: 1 in, 5 out]
        n451 = local read "Grain 1"() -> (w684:T2)
        n452 = call "Load Structure in VESTA.vi"("Vesta .exe Location"="Vesta .exe Location", "Atomic Structure"=w684) -> ()  [unwired: 10 in]
      }
      event "Load G2 VESTA": Value Change {
        n453 = event-data() -> ()  [unwired: 1 in, 5 out]
        n454 = local read "Vesta .exe Location"() -> (w685:path)
        n455 = local read "Grain 2"() -> (w686:T2)
        n456 = call "Load Structure in VESTA.vi"("Vesta .exe Location"=w685, "Atomic Structure"=w686) -> ()  [unwired: 10 in]
      }
      event "Load GB VESTA": Value Change {
        n457 = event-data() -> ()  [unwired: 1 in, 5 out]
        n458 = local read "Vesta .exe Location"() -> (w687:path)
        n459 = local read "Grain Boundary"() -> (w688:T2)
        n460 = call "Load Structure in VESTA.vi"("Vesta .exe Location"=w687, "Atomic Structure"=w688) -> ()  [unwired: 10 in]
      }
      event "Setup Camera": Value Change {
        n461 = event-data() -> ()  [unwired: 1 in, 5 out]
        n462 = local read "Grain Boundary"() -> (w704:T2)
        n463 = local read "Zoom Scale"() -> (w693:dbl)
        n464 = Unbundle By Name(w704) -> ("Lattice vector a"=w699:dbl[], "Lattice vector b"=w700:dbl[], "Lattice vector c"=w694:dbl[])
        n465 = Negate(x=w699) -> (-x=w701:dbl[])
        n466 = Array To Cluster(array=w700) -> (cluster=w690:T24)
        n467 = Compound Arithmetic op=ADD(w699, w700, w694) -> (w696:dbl[])
        n468 = Multiply(x=w701, y=2.0 ("Numeric")) -> (x*y=w703:dbl[])
        n469 = Divide(x=w696, y=2.0) -> (x/y=w697:dbl[])
        n470 = control-ref of="Grain Boundary Render"() -> (w689:refnum<vi>)
        n471 = Array To Cluster(array=w703) -> (cluster=w692:cluster{"[0]":dbl, "[1]":dbl, "[2]":dbl})
        n472 = Multiply(x=w697, y=w693) -> (x*y=w698:dbl[])
        n473 = Array To Cluster(array=w698) -> (cluster=w691:cluster{"[0]":dbl, "[1]":dbl, "[2]":dbl})
        n474 = invoke on="Invoke Node" class="SceneGraphDisp (strict)" method="Setup Camera"(reference=w689, "Camera Position"=w692, "Target"=w691, "Up Direction"=w690) -> ()  [unwired: 2 in, 6 out]
      }
    }
  }
  n475 = disable-structure shown="Enabled" {
    frame Disabled {
      n476 = local write "Conventional Unit Cell"(T2 {"Structure Name"="CdTe", "Lattice vector a"=[6.615785553057252, 0.0, 0.0], "Lattice vector b"=[0.0, 6.615785553057252, 0.0], "Lattice vector c"=[0.0, 0.0, 6.615785553057252], "Atoms Array"=[{"Atom Name"="Cd", "Positions (Direct)"=[[0.0, 0.0, 0.0], [0.0, 0.5, 0.5], [0.5, 0.0, 0.5], [0.5, 0.5, 0.0]], "Positions (Cartesian)"=[[0.0, 0.0, 0.0], [0.0, 3.307892776528626, 3.307892776528626], [3.307892776528626, 0.0, 3.307892776528626], [3.307892776528626, 3.307892776528626, 0.0]]}, {"Atom Name"="Te", "Positions (Direct)"=[[0.25, 0.25, 0.25], [0.75, 0.75, 0.25], [0.75, 0.25, 0.75], [0.25, 0.75, 0.75]], "Positions (Cartesian)"=[[1.653946388264313, 1.653946388264313, 1.653946388264313], [4.96183916479294, 4.96183916479294, 1.653946388264313], [4.96183916479294, 1.653946388264313, 4.96183916479294], [1.653946388264313, 4.96183916479294, 4.96183916479294]]}], "# of atoms"=8} ("Structure")) -> ()
    }
    frame Enabled {
    }
  }
  n477 = call <vilib>:"Create Object.vi"("Name"="Base") -> ("Scene:New Object"=→"Grain 2 Object":refnum<vi>)  [unwired: 1 in, 9 out]
  n478 = call <vilib>:"Create Object.vi"("Name"="Base") -> ("Scene:New Object"=→"Grain 1 Object":refnum<vi>)  [unwired: 1 in, 9 out]
  n479 = call <vilib>:"Create Object.vi"("Name"="Base") -> ("Scene:New Object"=→"Grain Boundary Object":refnum<vi>)  [unwired: 1 in, 9 out]
  n480 = local read "Conventional Unit Cell"() -> (w2:T2)
  n481 = Unbundle By Name(w2) -> ("Lattice vector a"=w3:dbl[])
  n482 = Square(x=w3) -> (x^2=w4:dbl[])
  n483 = Add Array Elements(numeric array=w4) -> (sum=w5:dbl)
  n484 = Square Root(x=w5) -> (sqrt(x)=→"Lattice Parameter":dbl)
